vi "BurstVIEW Analysis.vi"() -> ()   [LabVIEW 2017]
uses:
  <vilib>/Utility/config.llb/Config Data RefNum.ctl
  Application/Solution Package/Polarity.ctl
  Application/Solution Package/Minhee Analysis/Minhee analysis parameter_new.ctl
  Application/Solution Package/Data type_new.ctl
  <vilib>/Utility/sysdir.llb/System Directory Type.ctl
  <vilib>/Utility/miscctls.llb/LVRowAndColumnTypeDef.ctl
  <vilib>/Analysis/3filter.llb/Savitzky-Golay Filter (DBL).vi
  <vilib>/Utility/file.llb/Write Delimited Spreadsheet (DBL).vi
  <vilib>/Utility/file.llb/Write Delimited Spreadsheet (string).vi
  <vilib>/Analysis/NI_AALBase.lvlib
  <vilib>/Utility/config.llb/NI_LVConfig.lvlib
panel:
  out "Begin (sec)":string caption="String"
  out "End (sec)":string caption="String"
  out "Frequency":string caption="String"
  out "r^2 =":string caption="String"
  out "Decay t (ms)":string caption="String"
  out "Exponential \ncurve fitting":string
  out "History log":string
  in  "Event Detection Parameter":cluster{"Minimum amplitude":dbl, "Shape":T1}={"Minimum amplitude"=10.0, "Shape"=0} {"Shape" items=["Negative-going", "Positive-going"]}
  in  "Smoothing Parameters":T2={"Polynomial order"=3, "Side points"=35}
  out "Averaged Amplitude":sgl[](graph)
  out "StateFileRefnum":T3
  out "Event":cluster{dbl[], dbl[]}[](graph)
  out "Holding Current":sgl[](graph)
  out "Frequency 2":string caption="String"
  out "Number of event":i32[](graph)
  out "Event # 2":string caption="String"
  out "IEI (sec)  2":string caption="String"
  out "Amplitude 2":string caption="String"
  out "Event #":string caption="String"
  out "IEI (sec)":string caption="String"
  out "Amplitude (pA)":string caption="String"
  in  "Event Num":i16=4 min=0 max=42 step=1
  in  "Sweep Num":u16 max=16 step=1
  out "Event table":string[][](table)
  out "Whole trace":cluster{dbl[], "X":sgl[]}[](graph)
  # "Sweep info."
  # "Event table"
  # "Event detection parameters"
  # "Smoothing parameters"
  # "Result table"
  # "Event #"
  # "Amplitude (pA)"
  # "Total"
  # "IEI (sec)"
  # "Frequency (Hz)"
  # "Event #"
  # "Amplitude (pA)"
  # "IEI (sec)"
  # "Frequency (Hz)"
  # "Selected"
  # "Event search"
  # "Begin (sec)"
  # "End (sec)"
  # "Event"
  # "Sweep"
  # "Sweep"
  # "Log"
  # "(pA)"
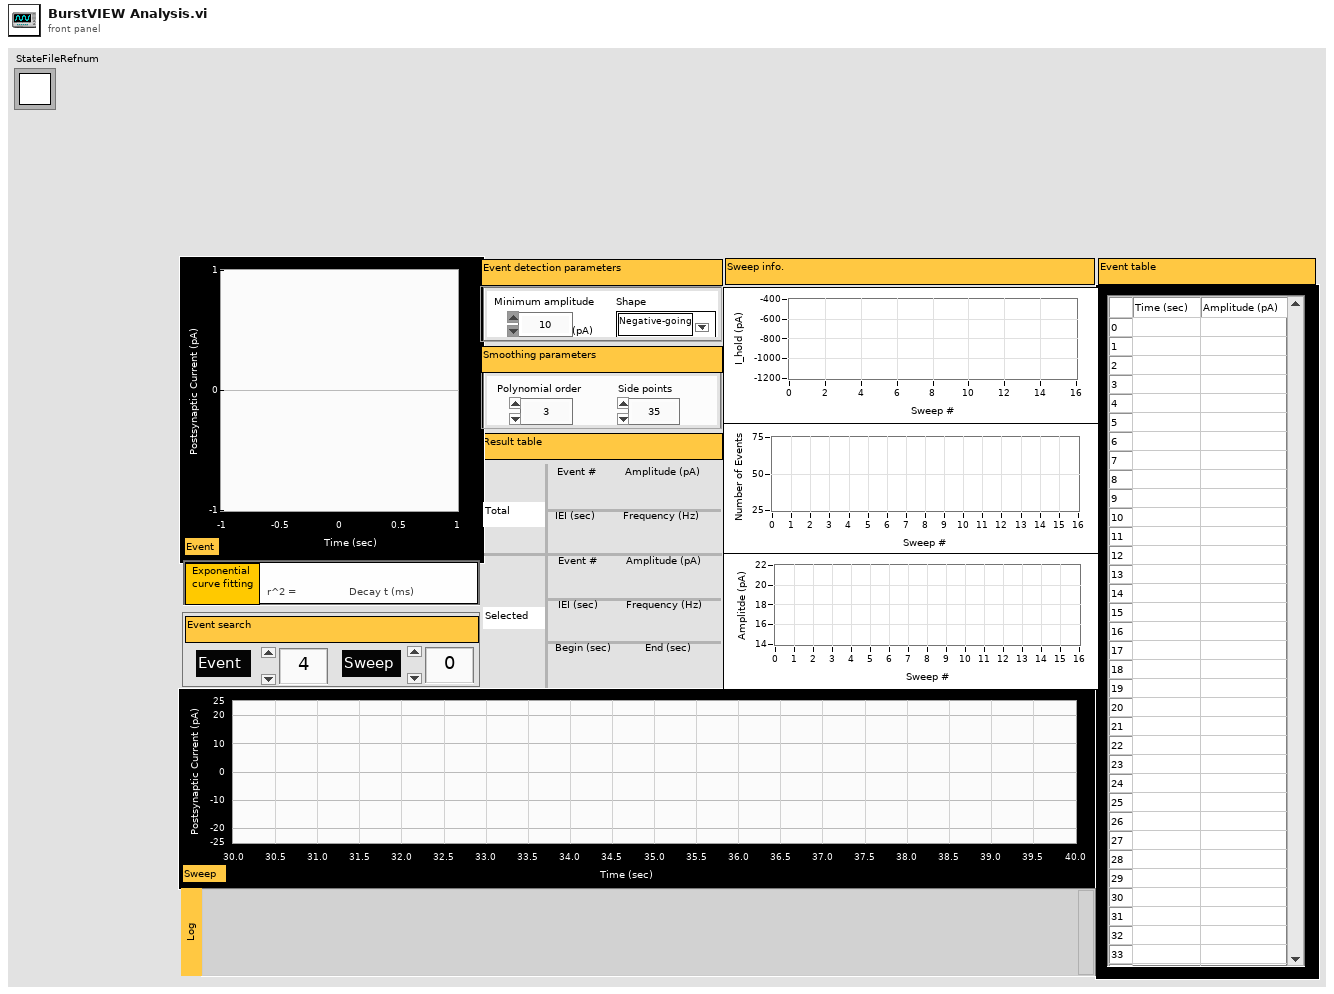
[diagram p1: front panel]
types:
  T1 = typedef "Polarity.ctl" = u16
  T2 = cluster{"Polynomial order":i32, "Side points":i32}
  T3 = typedef "NI_LVConfig.lvlib/Config Data RefNum.ctl" = refnum<k1>
  T4 = enum32{"Invalid", "Standard", "Closed", "Hidden", "Minimized", "Maximized"}
  T5 = enum32{"invalid app kind", "Development System", "Run Time System", "Student Edition", "Embedded LabVIEW", "Evaluation", "Custom"}
  T6 = enum16{"Linear", "Polynomial", "Exponential", "Power"}
  T7 = typedef "Minhee analysis parameter_new.ctl" = cluster{"File":cluster{"File Path":path, "File Name":string, "Total Length":i32, "Trial Length (ms)":dbl, "Sweep Number":dbl, "Sampling rate":dbl, "Data type":T8}, "Smoothing":cluster{"Polynomial order":i32, "Side points":i32}, "Event Detection ":cluster{"Event threshold (amplitude)":dbl, "Polarity":T1}, "Screening":cluster{"Screening threshold (dV/dt)":dbl, " * SD":dbl}}
  T8 = typedef "Data type_new.ctl" = u16
  T9 = cluster{"Core":cluster{"Current VI Reference":refnum<vi>, "Close Panel on Exit?":bool}, "Your Boolean data":bool, "Parameters":T7, "Whole trace (2D)":sgl[][], "Result":cluster{"Sweep Traces (2D)":cluster{sgl[], "X":sgl[]}[][], "Detected Events (1D)":cluster{sgl[][]}[], "Final Baseline":cluster{sgl[][]}[]}, "Running Sweep Num":i32, "Aborted?":bool, "Sweep Info":cluster{"Holding Current":sgl[], "Averaged Amplitude":sgl[], "Number of event":i32[]}, "Number of Event to select":i32, "Sweep Num":u16, "Event Num":i16, "Trace to display":u16, "History log":string, "Summary table":cluster{"Total":cluster{"Event Num":string, "Amplitude":string, "ISI":string, "Frequency":string}, "Selected":cluster{"Event Num":string, "Amplitude":string, "ISI":string, "Frequency":string, "Begin (sec)":string, "End (sec)":string}}, "Smoothing Parameters (1D)":cluster{"Polynomial order":i32, "Side points":i32}[], "Final Data":sgl[][], "Whole Trace selection":u16}
  T10 = cluster{"Polynomial order":i32, "Side points":i32}[]
  T11 = cluster{"Total":cluster{"Event Num":string, "Amplitude":string, "ISI":string, "Frequency":string}, "Selected":cluster{"Event Num":string, "Amplitude":string, "ISI":string, "Frequency":string, "Begin (sec)":string, "End (sec)":string}}
  T12 = cluster{"Sweep Traces (2D)":cluster{sgl[], "X":sgl[]}[][], "Detected Events (1D)":cluster{sgl[][]}[], "Final Baseline":cluster{sgl[][]}[]}
  T13 = cluster{"Holding Current":sgl[], "Averaged Amplitude":sgl[], "Number of event":i32[]}
  T14 = cluster{"Current VI Reference":refnum<vi>, "Close Panel on Exit?":bool}
  T15 = cluster{"Total":cluster{"Event Num":string, "Amplitude":string, "ISI":string, "Frequency":string}, "Selected":cluster{"Event Num":string, "Amplitude":string, "ISI":string, "Frequency":string, "Frequency 2":string, "Frequency 3":string}}
  T16 = typedef "System Directory Type.ctl" = i32
  T17 = typedef "LVRowAndColumnTypeDef.ctl" = cluster{"Row":i32, "Column":i32}
  T18 = cluster{"Event threshold (amplitude)":dbl, "Polarity":T1}
  T19 = cluster{"File Path":path, "Cell ID":string, "File Name":string, "Total Length":i32, "Trial Length (ms)":dbl, "Sweep Number":dbl, "Sampling rate":dbl}
  T20 = typedef "File Parameters.ctl" = cluster{"File path":path, "File name":string, "Total Length":i32, "Trial Length (ms)":i32, "Sweep Number":i32, "Sampling rate":dbl}
  T21 = cluster{"Sampling rate (Hz)":dbl, "Sweep duration (sec)":dbl, "Unit (A or pA)":u16, "Baseline Offset (pA)":dbl}
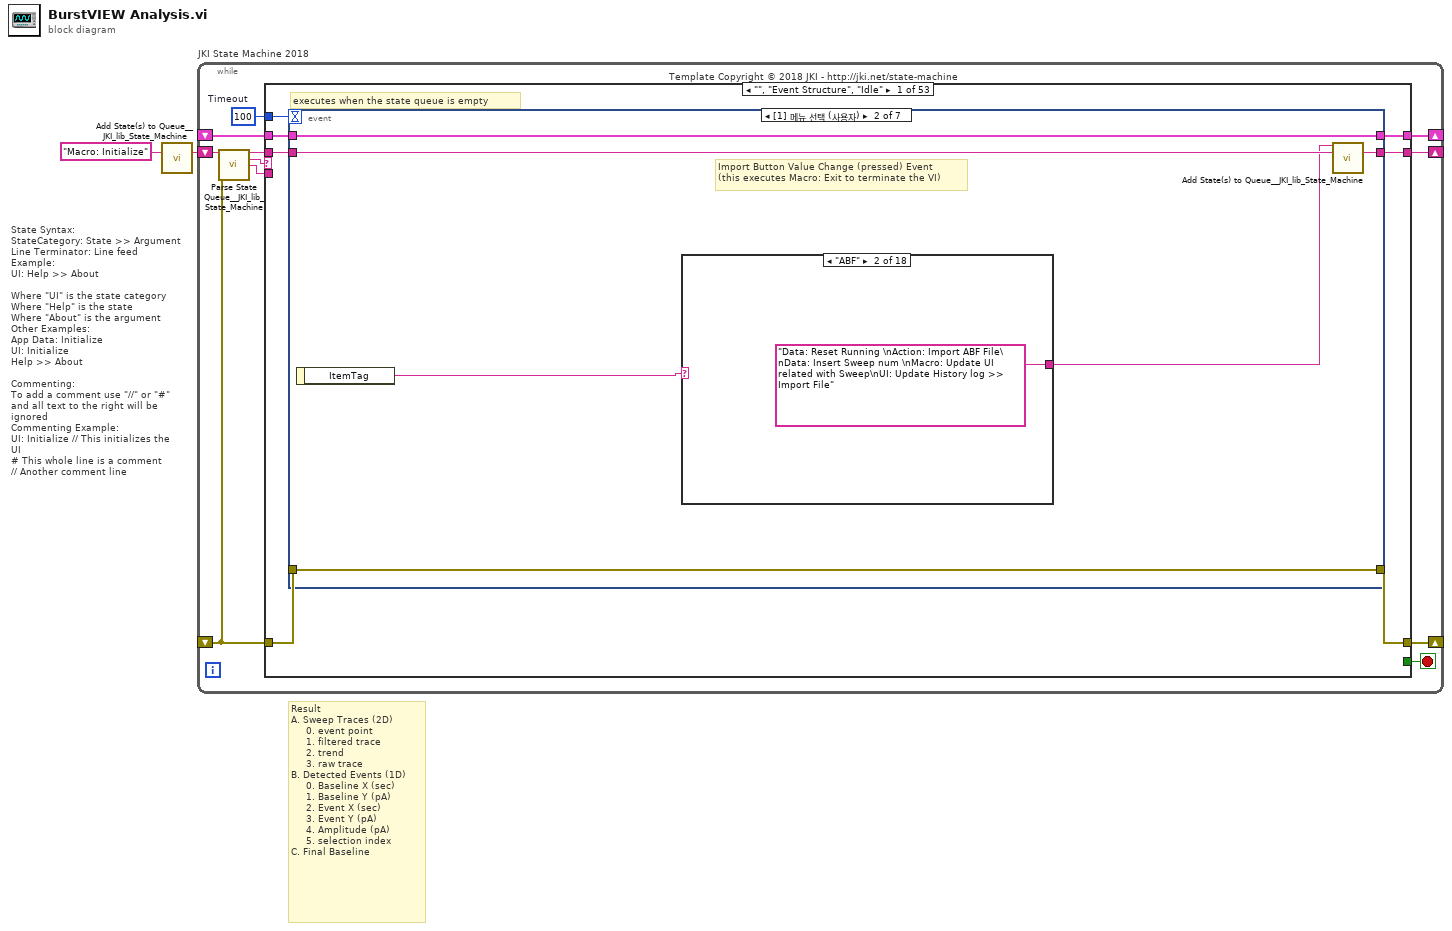
[diagram p0: block diagram]
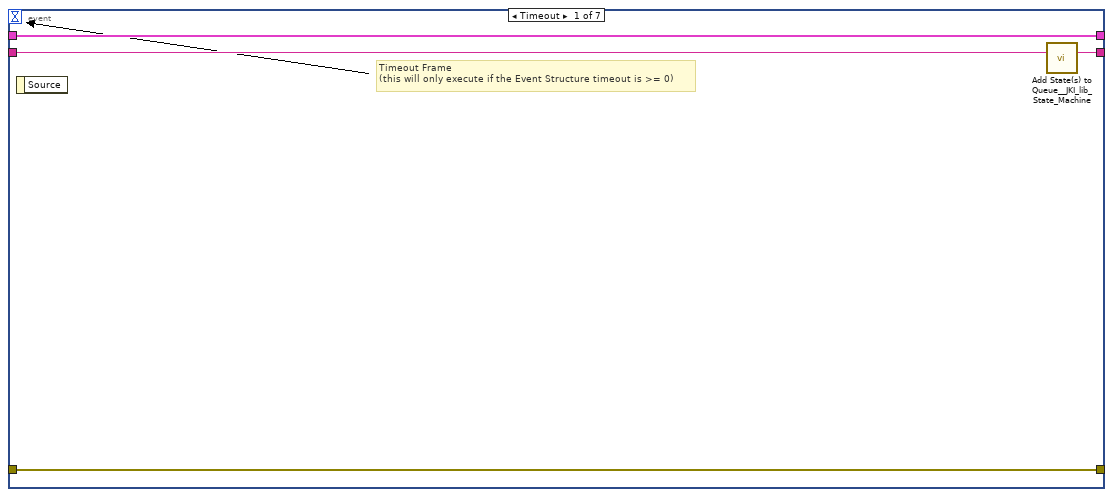
[diagram p2: hidden frame]
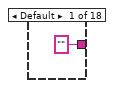
[diagram p3: hidden frame]
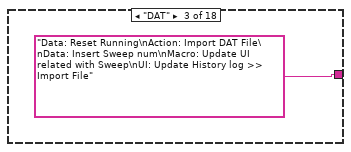
[diagram p4: hidden frame]
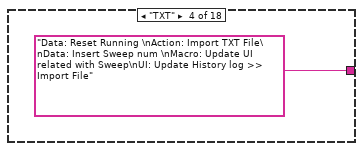
[diagram p5: hidden frame]
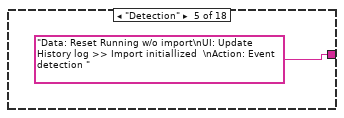
[diagram p6: hidden frame]
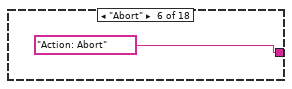
[diagram p7: hidden frame]
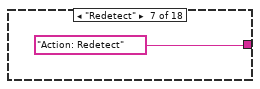
[diagram p8: hidden frame]
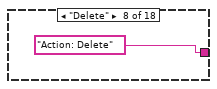
[diagram p9: hidden frame]
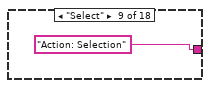
[diagram p10: hidden frame]
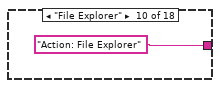
[diagram p11: hidden frame]
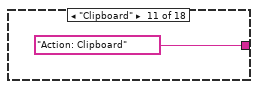
[diagram p12: hidden frame]
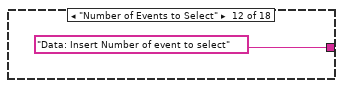
[diagram p13: hidden frame]
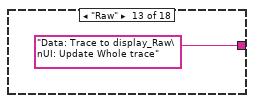
[diagram p14: hidden frame]
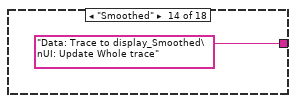
[diagram p15: hidden frame]
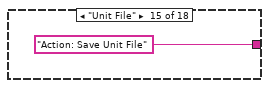
[diagram p16: hidden frame]
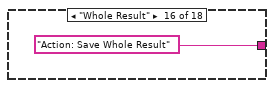
[diagram p17: hidden frame]
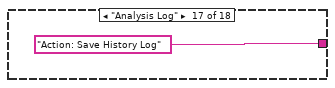
[diagram p18: hidden frame]
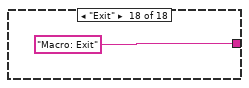
[diagram p19: hidden frame]
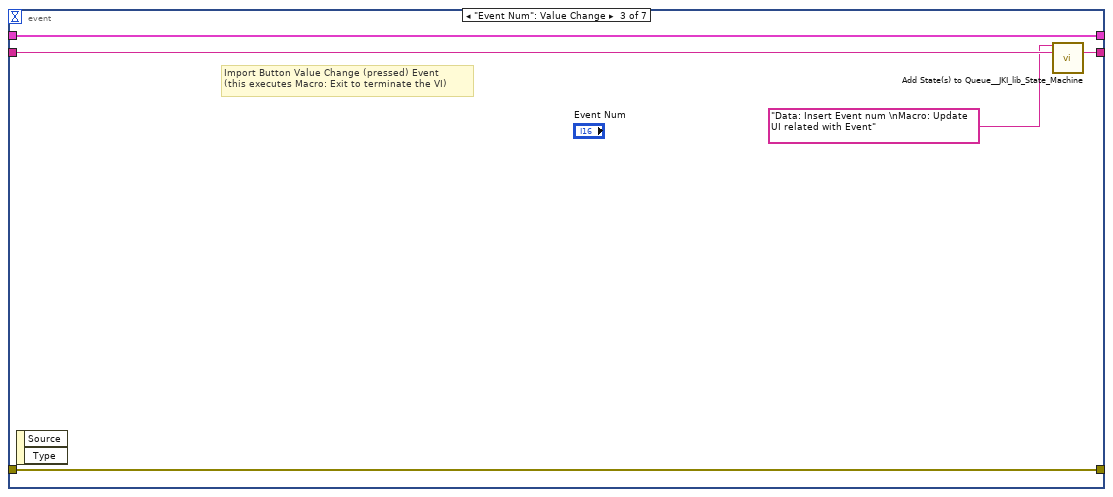
[diagram p20: hidden frame]
diagram:
  # "Result\nA. Sweep Traces (2D)\n     0. event point\n     1. filtered trace\n     2. trend\n     3. raw trace\nB. Detected Events (1D)\n     0. Baseline X (sec)\n     1. Baseline Y (pA)\n     2. Event X (sec)\n     3. Event Y (pA)\n     4. Amplitude (pA)\n     5. selection index\nC. Final Baseline"
  # "State Syntax:\nStateCategory: State >> Argument\nLine Terminator: Line feed\nExample:\nUI: Help >> About\n\nWhere \"UI\" is the state category\nWhere \"Help\" is the state\nWhere \"About\" is the argument\nOther Examples:\nApp Data: Initialize\nUI: Initialize\nHelp >> About\n\nCommenting:\nTo add a comment use \"//\" or \"#\" and all text to the right will be ignored\nCommenting Example:\nUI: Initialize // This initializes the UI\n# This whole line is a comment\n// Another comment line"
  n1 = call <vilib>:"Add State(s) to Queue__JKI_lib_State_Machine.vi"("State(s) in (\"\")"="Macro: Initialize") -> ("States Out"=w2:string)  [unwired: 14 in]
  n2 = while "JKI State Machine 2018" {
    shift-right: [w6] -> _
    shift-left: _ -> [w3]
    shift-right: [w9] -> _
    shift-left: _ -> [w4]
    shift-right: [w8] -> _
    shift-left: w2 -> [w10]
    stop <- w7 stop-if-true
    w5 = 100  # Timeout
    # "Template Copyright © 2018 JKI - http://jki.net/state-machine"
    n3 = call <vilib>:"Parse State Queue__JKI_lib_State_Machine.vi"("State Queue"=w10, "Error In (no error)"=w4) -> ("Remaining States"=w12:string, "Current State"=w13:string, "Arguments"=w11:string)  [unwired: 11 in]
    n4 = case shown="\"\", \"Event Structure\", \"Idle\"" w13 {
      selector: w13 -> [_ _ w79 _ _ _ _ _ _ _ _ _ _ _ _ _ _ _ _ _ _ _ _ _ _ _ _ _ _ _ _ _ _ _ _ _ _ _ _ _ _ _ _ _ _ _ _ _ _ _ _ _ _]
      tunnel: w12 -> [w20 w78 w83 w102 w108 w114 w124 w147 w161 w173 w182 w188 w194 w200 w206 w212 w218 w224 w232 w238 w242 w260 w284 w336 w375 w384 w400 w427 w453 w463 w478 w576 w587 w656 w661 w666 w671 w676 w686 w697 w717 w737 w758 w819 w829 w860 w882 w938 w958 w968 w985 w996 w1005]
      tunnel: w11 -> [_ _ _ _ _ _ _ _ _ _ _ _ _ _ _ _ _ _ _ _ _ _ _ _ _ _ _ _ _ _ w472 w571 w581 _ _ _ _ _ _ _ _ _ _ _ _ _ _ _ _ _ _ _ _]
      tunnel: w3 -> [w18 w75 w81 w95 w105 w112 w121 _ w158 w170 w179 w185 w191 w197 w203 w209 w215 w221 w230 w233 w239 w248 w273 w334 w373 w381 w397 w417 w450 w461 w475 w574 w583 w653 w658 w663 w668 w673 w683 w694 w714 w735 w754 w804 w826 w847 w880 w904 w954 w965 w982 w993 w1002]
      tunnel: [w17 w76 w85 w99 errorcluster {"status"=FALSE, "code"=0, "source"=""} ("error out") w111 w122 w126 w159 w171 w180 w186 w192 w198 w204 w210 w216 w222 w225 w234 w240 w249 w282 w324 w339 w382 w398 w425 w451 w454 w476 w572 w584 w654 w659 w664 w669 w674 w684 w695 w706 w733 w746 w812 w827 w830 w871 w935 w955 w966 w969 w990 w999] -> w9
      tunnel: w4 -> [w16 w76 w84 w99 w104 w111 w122 w127 w159 w171 w180 w186 w192 w198 w204 w210 w216 w222 w226 w235 w240 w246 w267 w325 w340 w382 w398 w425 w451 w455 w476 w573 w585 w654 w659 w664 w669 w674 w684 w695 w699 w728 w756 w813 w827 w831 w872 w935 w956 w966 w970 w991 w1000]
      tunnel: [w19 w77 w82 w101 w107 w113 w123 w146 w160 w172 w181 w187 w193 w199 w205 w211 w217 w223 w231 w237 w241 w259 w283 w335 w374 w383 w399 w426 w452 w462 w477 w575 w586 w655 w660 w665 w670 w675 w685 w696 w716 w736 w757 w818 w828 w859 w881 w937 w957 w967 w984 w995 w1004] -> w8
      tunnel: [_ _ _ _ _ w109 _ _ _ _ _ _ _ _ _ _ _ _ _ _ _ _ _ _ _ _ _ _ _ _ _ _ _ _ _ _ _ _ _ _ _ _ _ _ _ _ _ _ _ _ _ _ _] -> w7
      tunnel: [w15 w75 w81 w100 w105 w112 w121 w145 w157 w169 w178 w184 w190 w196 w202 w208 w214 w220 w229 w233 w239 w248 w273 w334 w373 w381 w397 w416 w450 w461 w474 w574 w583 w653 w658 w663 w668 w673 w683 w694 w713 w734 w753 w803 w825 w846 w879 w903 w954 w965 w982 w993 w1002] -> w6
      tunnel: w5 -> [w14 _ _ _ _ _ _ _ _ _ _ _ _ _ _ _ _ _ _ _ _ _ _ _ _ _ _ _ _ _ _ _ _ _ _ _ _ _ _ _ _ _ _ _ _ _ _ _ _ _ _ _ _]
      frame "", "Event Structure", "Idle" {
        # "executes when the state queue is empty"
        n5 = event shown="[1] 메뉴 선택 (사용자)" {
          selector: _ -> [_ _ _ _ _ _ _]
          dyn-events: _ -> [_ _ _ _ _ _ _]
          timeout: w14 -> [_ _ _ _ _ _ _]
          tunnel: w20 -> [w24 w30 w53 w58 w63 w68 w74]
          tunnel: [w23 w29 w52 w57 w62 w67 w73] -> w19
          tunnel: w18 -> [w21 w27 w49 w54 w59 w64 w71]
          tunnel: [w22 w28 w51 w56 w61 w66 w72] -> w17
          tunnel: w16 -> [w22 w28 w51 w56 w61 w66 w72]
          tunnel: [w21 w27 w49 w54 w59 w64 w71] -> w15
          event Timeout {
            # "Timeout Frame\n(this will only execute if the Event Structure timeout is >= 0)"
            n6 = event-data() -> ()  [unwired: 1 in, 1 out]
            n7 = call <vilib>:"Add State(s) to Queue__JKI_lib_State_Machine.vi"("State(s) in (\"\")"=w24) -> ("States Out"=w23:string)  [unwired: 14 in]
          }
          event Menu Selection (User) {
            # "Import Button Value Change (pressed) Event\n(this executes Macro: Exit to terminate the VI)"
            n8 = event-data() -> ("ItemTag"=w25:string)  [unwired: 1 in]
            n9 = case shown="\"ABF\"" w25 {
              tunnel: ["" "Data: Reset Running \nAction: Import ABF File\nData: Insert Sweep num \nMacro: Update UI related with Sweep\nUI: Update History log >> Import File" "Data: Reset Running\nAction: Import DAT File\nData: Insert Sweep num\nMacro: Update UI related with Sweep\nUI: Update History log >> Import File" "Data: Reset Running \nAction: Import TXT File\nData: Insert Sweep num \nMacro: Update UI related with Sweep\nUI: Update History log >> Import File" "Data: Reset Running w/o import\nUI: Update History log >> Import initiallized  \nAction: Event detection " "Action: Abort" "Action: Redetect" "Action: Delete" "Action: Selection" "Action: File Explorer" "Action: Clipboard" "Data: Insert Number of event to select" "Data: Trace to display_Raw\nUI: Update Whole trace" "Data: Trace to display_Smoothed\nUI: Update Whole trace" "Action: Save Unit File" "Action: Save Whole Result" "Action: Save History Log" "Macro: Exit"] -> w26
              frame Default {
              }
              frame "ABF" {
              }
              frame "DAT" {
              }
              frame "TXT" {
              }
              frame "Detection" {
              }
              frame "Abort" {
              }
              frame "Redetect" {
              }
              frame "Delete" {
              }
              frame "Select" {
              }
              frame "File Explorer" {
              }
              frame "Clipboard" {
              }
              frame "Number of Events to Select" {
              }
              frame "Raw" {
              }
              frame "Smoothed" {
              }
              frame "Unit File" {
              }
              frame "Whole Result" {
              }
              frame "Analysis Log" {
              }
              frame "Exit" {
              }
            }
            n10 = call <vilib>:"Add State(s) to Queue__JKI_lib_State_Machine.vi"("State(s) in Front (\"\")"=w26, "State(s) in (\"\")"=w30) -> ("States Out"=w29:string)  [unwired: 13 in]
          }
          event "Event Num": Value Change {
            # "Import Button Value Change (pressed) Event\n(this executes Macro: Exit to terminate the VI)"
            n11 = event-data() -> ()  [unwired: 1 in, 2 out]
            n12 = call <vilib>:"Add State(s) to Queue__JKI_lib_State_Machine.vi"("State(s) in Front (\"\")"="Data: Insert Event num \nMacro: Update UI related with Event", "State(s) in (\"\")"=w53) -> ("States Out"=w52:string)  [unwired: 13 in]
          }
          event "Sweep Num": Value Change {
            # "Import Button Value Change (pressed) Event\n(this executes Macro: Exit to terminate the VI)"
            n13 = event-data() -> ()  [unwired: 1 in, 2 out]
            n14 = call <vilib>:"Add State(s) to Queue__JKI_lib_State_Machine.vi"("State(s) in Front (\"\")"="Data: Insert Sweep num \nMacro: Update UI related with Sweep \nMacro: Update UI related with Event", "State(s) in (\"\")"=w58) -> ("States Out"=w57:string)  [unwired: 13 in]
          }
          event "Event Detection Parameter.Minimum amplitude": Value Change {
            # "Import Button Value Change (pressed) Event\n(this executes Macro: Exit to terminate the VI)"
            n15 = event-data() -> ()  [unwired: 1 in, 2 out]
            n16 = call <vilib>:"Add State(s) to Queue__JKI_lib_State_Machine.vi"("State(s) in Front (\"\")"="Data: Insert Event detection parameters", "State(s) in (\"\")"=w63) -> ("States Out"=w62:string)  [unwired: 13 in]
          }
          event "Smoothing Parameters.Polynomial order", "Smoothing Parameters.Side points": Value Change {
            # "Import Button Value Change (pressed) Event\n(this executes Macro: Exit to terminate the VI)"
            n17 = event-data() -> ()  [unwired: 1 in, 2 out]
            n18 = call <vilib>:"Add State(s) to Queue__JKI_lib_State_Machine.vi"("State(s) in Front (\"\")"="Data: Insert Smoothing parameters", "State(s) in (\"\")"=w68) -> ("States Out"=w67:string)  [unwired: 13 in]
          }
          event Panel Close? {
            # "Discard the event because we'll close the front panel ourselves in Macro: Exit"
            # "Close Panel button (pressed) Event\n(this executes Macro: Exit to terminate the VI)"
            n19 = event-data() -> ()  [unwired: 1 in, 1 out]
            n20 = call <vilib>:"Add State(s) to Queue__JKI_lib_State_Machine.vi"("State(s) in Front (\"\")"="Macro: Exit", "State(s) in (\"\")"=w74) -> ("States Out"=w73:string)  [unwired: 13 in]
            n21 = event-data("Discard?"=TRUE) -> ()  [unwired: 1 in, 1 out]
          }
        }
      }
      frame "---------- Core ----------" {
        # "Do not put any code in this frame.\n(it is a separator no-op)"
        n22 = call <vilib>:"Add State(s) to Queue__JKI_lib_State_Machine.vi"("State(s) in (\"\")"=w78) -> ("States Out"=w77:string)  [unwired: 14 in]
      }
      frame Default {
        w88 = 42 items=["No error", "Argument error", "Memory is full", "Out of zone", "End of file", "File already open", "Generic file I/O error", "File not found", "File permission error", "Disk is full", "Duplicate path", "Too many files open", "System feature not enabled", "Resource file not found", "Cannot add resource", "Resource not found", "Image not found", "Image memory error", "Pen does not exist", "Config type invalid", "Config token not found", "Config parse error", "Config memory error", "Bad external code format", "Bad external code offset", "External code not present", "Null window", "Destroy window error", "Null menu", "Print aborted", "Bad print record", "Print driver error", "Windows error during printing", "Memory error during printing", "Print dialog error", "Generic print error", "Invalid device refnum", "Device not found", "Device parameter error", "Device unit error", "Cannot open device", "Device call aborted", "Generic error", "Cancelled by user", "Object ID too low", "Object ID too high", "Object not in heap", "Unknown heap", "Unknown object (invalid DefProc)", "Unknown object (DefProc not in table)", "Message out of range", "Invalid (null) method", "Unknown message", "Manager call not supported", "Bad address", "Network operation in progress", "Network operation timed out", "Connection is busy", "Network attribute not supported", "Network error", "Address in use", "System out of memory", "Connection aborted", "Connection refused", "Not connected", "Already connected", "Connection closed", "Initialization error (interapplication manager)", "Bad occurrence", "Wait on unbound occurrence handler", "Occurrence queue overflow", "Datalog type conflict", "Unused", "Unrecognized type (interapplication manager)", "Memory corrupt", "Failed to make temporary DLL", "Old CIN version", "Drag socket not found", "Failed to load drop-object", "Failed to register OLE object", "Failed to release OLE object", "Format specifier type mismatch", "Unknown format specifier", "Too few format specifiers", "Too many format specifiers", "Scan failed", "Newer CIN version", "Error converting to variant", "Runtime menu error", "Password tampered", "Variant attribute not found", "Incompatible variant data type", "Event data is not available", "Event Store is not present", "Occurrence is not found", "Event Queue is not created", "Event info is not available", "Refnum passed is NULL", "Error retrieving Class GUID", "Error retrieving CoClass GUID", "Error retrieving TypeLib GUID.", "Bad built application magic bytes.", "Specific driver is different from the specific driver associated with the Logical Name.", "There is no session opened to the class driver.", "Max Error", "MAX - Error with config objects", "MAX - Error loading configuration", "MAX - Group not supported"]
        # "Current State"
        # "Do not delete, rename, or modify this frame.\n(this is used to capture unhandled states and typos)"
        # "Handle mistyped state name (developer tool)"
        n23 = Format Into String(format string="Software Exception: Unhandled State \"%s\"." ("message"), error in=w84, w79) -> (resulting string=w87:string, error out=w86:errorcluster)  [unwired: 1 in]
        n24 = call <vilib>:"Error Cluster From Error Code.vi"("show call chain? (False)"=TRUE, "error in (no error)"=w86, "error message (\"\")"=w87, "error code (0)"=w88) -> ("error out"=w85:errorcluster)  [unwired: 5 in]
        n25 = call <vilib>:"Add State(s) to Queue__JKI_lib_State_Machine.vi"("State(s) in (\"\")"=w83) -> ("States Out"=w82:string)  [unwired: 14 in]
      }
      frame "Initialize Core Data" {
        # "Do not delete, rename, or modify this frame.\n(this is used to determine panel behavior on exit)"
        # "originally closed?"
        # "exe?"
        # "If panel starts closed or is an EXE, then close it when we exit"
        n26 = property class="VI"() -> ("FP.State"=w92:T4)  [unwired: 2 in, 2 out]
        n27 = property class="App"() -> ("App.Kind"=w98:T5)  [unwired: 2 in, 2 out]
        n28 = control-ref of="Current VI Reference"() -> (w93:refnum<vi>)
        n29 = Equal?(x=w92, y=T4."Closed" ("Front Panel Window:State")) -> (x = y?=w90:bool)
        n30 = Equal?(x=w98, y=T5."Run Time System" ("Application:Kind")) -> (x = y?=w96:bool)
        n31 = Or(x=w90, y=w96) -> (x .or. y?=w94:bool)
        n32 = Bundle By Name(cluster=w95, "Core.Current VI Reference"=w93, "Core.Close Panel on Exit?"=w94) -> (w100:T9)
        n33 = call <vilib>:"Add State(s) to Queue__JKI_lib_State_Machine.vi"("State(s) in (\"\")"=w102) -> ("States Out"=w101:string)  [unwired: 14 in]
      }
      frame "Error Handler" {
        # "Unhandled Error -- Display it"
        # "Handle any errors here.\nYou can also output any states to clean-up after errors occur"
        # "Clear error"
        n34 = call <vilib>:"General Error Handler.vi"("error in (no error)"=w104) -> ()  [unwired: 10 in, 5 out]
        n35 = call <vilib>:"Add State(s) to Queue__JKI_lib_State_Machine.vi"("State(s) in Front (\"\")"="/* Post Error States", "State(s) in (\"\")"=w108) -> ("States Out"=w107:string)  [unwired: 13 in]
      }
      frame "Exit" {
        # "Do not put any code in this frame.\n(No errors that occur here will be handled.)"
        n36 = flat-sequence {
          tunnel: [w115] -> w110
          tunnel: w110 -> [w120]
          tunnel: [w119] -> w109
          frame #0 {
            n37 = local read "StateFileRefnum"() -> (w115:T3)
            n38 = Current VI's Path ("Current VI's Path...")() -> (path=w116:path)
            n39 = Open VI Reference(vi path=w116) -> (vi reference=w117:refnum<vi>)  [unwired: 5 in, 1 out]
            n40 = call <userlib>:"SaveVIState.vi"("StateFileRefnum"=w115, "key"="StateKey", "VI Refnum"=w117) -> ()
          }
          frame #1 {
            w119 = TRUE ("write configuration file? (F)")
            n41 = call <vilib>:"Close Config Data.vi"("write file if changed (T)"=w119, "refnum"=w120) -> ()  [unwired: 8 in, 2 out]
          }
        }
        n42 = call <vilib>:"Add State(s) to Queue__JKI_lib_State_Machine.vi"("State(s) in (\"\")"=w114) -> ("States Out"=w113:string)  [unwired: 14 in]
      }
      frame "---------- Data ----------" {
        # "Do not put any code in this frame.\n(It is a separator no-op. You can make a copy of this frame to create a new Data frame)"
        n43 = call <vilib>:"Add State(s) to Queue__JKI_lib_State_Machine.vi"("State(s) in (\"\")"=w124) -> ("States Out"=w123:string)  [unwired: 14 in]
      }
      frame "Data: Initialize" {
        w125 = u16 0 items=["Imported", "Analyzed"]  # Whole Trace selection
        w131 = sgl[][] []  # Final Data
        w132 = T10 []  # Smoothing Parameters (1D)
        w133 = T11 {"Total"={"Event Num"="", "Amplitude"="", "ISI"="", "Frequency"=""}, "Selected"={"Event Num"="", "Amplitude"="", "ISI"="", "Frequency"="", "Begin (sec)"="", "End (sec)"=""}}  # Summary table
        w134 = ""  # History log
        w135 = u16 0 items=["Raw", "Smoothed"]  # Trace to display
        w136 = T12 {"Sweep Traces (2D)"=[], "Detected Events (1D)"=[], "Final Baseline"=[]}  # Result
        w129 = i16 0  # Event Num
        w130 = u16 0  # Sweep Num
        w137 = 200  # Number of Event to select
        w138 = T13 {"Holding Current"=[], "Averaged Amplitude"=[], "Number of event"=[]}  # Sweep Info
        w139 = FALSE  # Aborted?
        w140 = 0  # Running Sweep Num
        w141 = sgl[][] []  # Whole trace (2D)
        w142 = T7 {"File"={"File Path"=path "", "File Name"="", "Total Length"=0, "Trial Length (ms)"=0.0, "Sweep Number"=0.0, "Sampling rate"=0.0, "Data type"=0}, "Smoothing"={"Polynomial order"=3, "Side points"=20}, "Event Detection "={"Event threshold (amplitude)"=10.0, "Polarity"=0}, "Screening"={"Screening threshold (dV/dt)"=0.0, " * SD"=2.5}}  # Parameters
        w143 = T14 {"Current VI Reference"=refnum, "Close Panel on Exit?"=FALSE}  # Core
        w144 = TRUE  # Your Boolean data
        # "Result\nA. Sweep Traces (2D)\n     0. event point\n     1. filtered trace\n     2. trend\n     3. raw trace\nB. Detected Events (1D)\n     0. Baseline X (sec)\n     1. Baseline Y (pA)\n     2. Event X (sec)\n     3. Event Y (pA)\n     4. Amplitude (pA)\n     5. selection index\nC. Final Baseline"
        # "do not delete - used by framework"
        # "Data names and types of shift register data are defined by this bundle."
        # "Initialize the shift-register data, here.\n(data names are defined by what you wire into the bundle function)"
        n44 = property on="Sweep Num" class="DigNum (엄격한)"(error in=w127, "Value"=w130) -> (error out=w128:errorcluster)  [unwired: 1 in, 1 out]
        n45 = property on="Event Num" class="DigNum (엄격한)"(error in=w128, "Value"=w129) -> (error out=w126:errorcluster)  [unwired: 1 in, 1 out]
        n46 = Bundle("Core"=w143, "Your Boolean data"=w144, "Parameters"=w142, "Whole trace (2D)"=w141, "Result"=w136, "Running Sweep Num"=w140, "Aborted?"=w139, "Sweep Info"=w138, "Number of Event to select"=w137, "Sweep Num"=w130, "Event Num"=w129, "Trace to display"=w135, "History log"=w134, "Summary table"=w133, "Smoothing Parameters (1D)"=w132, "Final Data"=w131, "Whole Trace selection"=w125) -> (w145:T9)  [unwired: 1 in]
        n47 = call <vilib>:"Add State(s) to Queue__JKI_lib_State_Machine.vi"("State(s) in (\"\")"=w147) -> ("States Out"=w146:string)  [unwired: 14 in]
      }
      frame "Data: Reset Running" {
        w148 = u16 0 items=["Imported", "Analyzed"]  # Whole Trace selection
        w151 = T15 {"Total"={"Event Num"="", "Amplitude"="", "ISI"="", "Frequency"=""}, "Selected"={"Event Num"="", "Amplitude"="", "ISI"="", "Frequency"="", "Frequency 2"="", "Frequency 3"=""}}  # Summary table
        w152 = T12 {"Sweep Traces (2D)"=[], "Detected Events (1D)"=[], "Final Baseline"=[]}  # Result
        w154 = T13 {"Holding Current"=[], "Averaged Amplitude"=[], "Number of event"=[]}  # Sweep Info
        # "Do not put any code in this frame.\n(It is a separator no-op. You can make a copy of this frame to create a new Data frame)"
        n48 = Bundle By Name(cluster=w158, "Running Sweep Num"=0 ("Running Sweep #"), "Aborted?"=FALSE ("Aborted"), "Sweep Info"=w154, "Whole trace (2D)"=sgl[][] [], "Result"=w152, "Summary table"=w151, "Whole Trace selection"=w148) -> (w157:T9)
        n49 = local write "Whole trace"(cluster{sgl[], "X":sgl[]}[] [{[], "X"=[]}, {[], "X"=[]}, {[], "X"=[]}] ("Whole trace")) -> ()
        n50 = local write "Event"(cluster{sgl[], sgl[]}[] [{[], []}, {[], []}, {[], []}, {[], []}] ("Event trace")) -> ()
        n51 = call <vilib>:"Add State(s) to Queue__JKI_lib_State_Machine.vi"("State(s) in (\"\")"=w161) -> ("States Out"=w160:string)  [unwired: 14 in]
      }
      frame "Data: Reset Running w/o import" {
        w164 = T15 {"Total"={"Event Num"="", "Amplitude"="", "ISI"="", "Frequency"=""}, "Selected"={"Event Num"="", "Amplitude"="", "ISI"="", "Frequency"="", "Frequency 2"="", "Frequency 3"=""}}  # Summary table
        w165 = T12 {"Sweep Traces (2D)"=[], "Detected Events (1D)"=[], "Final Baseline"=[]}  # Result
        w166 = T13 {"Holding Current"=[], "Averaged Amplitude"=[], "Number of event"=[]}  # Sweep Info
        # "Do not put any code in this frame.\n(It is a separator no-op. You can make a copy of this frame to create a new Data frame)"
        n52 = Bundle By Name(cluster=w170, "Running Sweep Num"=0 ("Running Sweep #"), "Aborted?"=FALSE ("Aborted"), "Sweep Info"=w166, "Result"=w165, "Summary table"=w164) -> (w169:T9)
        n53 = local write "Whole trace"(cluster{sgl[], "X":sgl[]}[] [{[], "X"=[]}, {[], "X"=[]}, {[], "X"=[]}] ("Whole trace")) -> ()
        n54 = local write "Event"(cluster{sgl[], sgl[]}[] [{[], []}, {[], []}, {[], []}, {[], []}] ("Event trace")) -> ()
        n55 = call <vilib>:"Add State(s) to Queue__JKI_lib_State_Machine.vi"("State(s) in (\"\")"=w173) -> ("States Out"=w172:string)  [unwired: 14 in]
      }
      frame "Data: Insert inital parameters" {
        # "Do not put any code in this frame.\n(It is a separator no-op. You can make a copy of this frame to create a new Data frame)"
        n56 = local read "Event Detection Parameter"() -> (w175:cluster{"Minimum amplitude":dbl, "Shape":T1})
        n57 = local read "Smoothing Parameters"() -> (w174:T2)
        n58 = local read "Sweep Num"() -> (w177:u16)
        n59 = local read "Event Num"() -> (w176:i16)
        n60 = Bundle By Name(cluster=w179, "Sweep Num"=w177, "Event Num"=w176, "Parameters.Smoothing"=w174, "Parameters.Event Detection"=w175) -> (w178:T9)
        n61 = call <vilib>:"Add State(s) to Queue__JKI_lib_State_Machine.vi"("State(s) in (\"\")"=w182) -> ("States Out"=w181:string)  [unwired: 14 in]
      }
      frame "Data: Insert Sweep num" {
        # "Do not put any code in this frame.\n(It is a separator no-op. You can make a copy of this frame to create a new Data frame)"
        n62 = local read "Sweep Num"() -> (w183:u16)
        n63 = Bundle By Name(cluster=w185, "Sweep Num"=w183) -> (w184:T9)
        n64 = call <vilib>:"Add State(s) to Queue__JKI_lib_State_Machine.vi"("State(s) in (\"\")"=w188) -> ("States Out"=w187:string)  [unwired: 14 in]
      }
      frame "Data: Insert Event num" {
        # "Do not put any code in this frame.\n(It is a separator no-op. You can make a copy of this frame to create a new Data frame)"
        n65 = local read "Event Num"() -> (w189:i16)
        n66 = Bundle By Name(cluster=w191, "Event Num"=w189) -> (w190:T9)
        n67 = call <vilib>:"Add State(s) to Queue__JKI_lib_State_Machine.vi"("State(s) in (\"\")"=w194) -> ("States Out"=w193:string)  [unwired: 14 in]
      }
      frame "Data: Insert Event detection parameters" {
        # "Do not put any code in this frame.\n(It is a separator no-op. You can make a copy of this frame to create a new Data frame)"
        n68 = local read "Event Detection Parameter"() -> (w195:cluster{"Minimum amplitude":dbl, "Shape":T1})
        n69 = Bundle By Name(cluster=w197, "Parameters.Event Detection"=w195) -> (w196:T9)
        n70 = call <vilib>:"Add State(s) to Queue__JKI_lib_State_Machine.vi"("State(s) in (\"\")"=w200) -> ("States Out"=w199:string)  [unwired: 14 in]
      }
      frame "Data: Insert Smoothing parameters" {
        n71 = local read "Smoothing Parameters"() -> (w201:T2)
        n72 = Bundle By Name(cluster=w203, "Parameters.Smoothing"=w201) -> (w202:T9)
        n73 = call <vilib>:"Add State(s) to Queue__JKI_lib_State_Machine.vi"("State(s) in (\"\")"=w206) -> ("States Out"=w205:string)  [unwired: 14 in]
      }
      frame "Data: Trace to display_Raw" {
        # "Do not put any code in this frame.\n(It is a separator no-op. You can make a copy of this frame to create a new Data frame)"
        n74 = Bundle By Name(cluster=w209, "Trace to display"=u16 0) -> (w208:T9)
        n75 = call <vilib>:"Add State(s) to Queue__JKI_lib_State_Machine.vi"("State(s) in (\"\")"=w212) -> ("States Out"=w211:string)  [unwired: 14 in]
      }
      frame "Data: Trace to display_Smoothed" {
        # "Do not put any code in this frame.\n(It is a separator no-op. You can make a copy of this frame to create a new Data frame)"
        n76 = Bundle By Name(cluster=w215, "Trace to display"=u16 1) -> (w214:T9)
        n77 = call <vilib>:"Add State(s) to Queue__JKI_lib_State_Machine.vi"("State(s) in (\"\")"=w218) -> ("States Out"=w217:string)  [unwired: 14 in]
      }
      frame "Data: Whole trace selection" {
        # "Do not put any code in this frame.\n(It is a separator no-op. You can make a copy of this frame to create a new Data frame)"
        n78 = Bundle By Name(cluster=w221, "Whole Trace selection"=u16 1) -> (w220:T9)
        n79 = call <vilib>:"Add State(s) to Queue__JKI_lib_State_Machine.vi"("State(s) in (\"\")"=w224) -> ("States Out"=w223:string)  [unwired: 14 in]
      }
      frame "Data: Insert Number of event to select" {
        # "Do not put any code in this frame.\n(It is a separator no-op. You can make a copy of this frame to create a new Data frame)"
        n80 = call "Number of Events to Select"("error in (no error)"=w226) -> ("Number of Events"=w228:dbl, "error out"=w225:errorcluster)  [unwired: 16 in, 1 out]
        n81 = To Long Integer(number=w228) -> (32bit integer=w227:i32)
        n82 = Bundle By Name(cluster=w230, "Number of Event to select"=w227) -> (w229:T9)
        n83 = call <vilib>:"Add State(s) to Queue__JKI_lib_State_Machine.vi"("State(s) in (\"\")"=w232) -> ("States Out"=w231:string)  [unwired: 14 in]
      }
      frame "Data: Cleanup" {
        # "Cleanup any data and references, here.\n(this is called automatically, by the Macro: Exit)"
        n84 = Unbundle By Name(w233) -> ("Core.Current VI Reference"=w236:refnum<vi>)
        n85 = Close Reference(reference=w236, error in (no error)=w235) -> (error out=w234:errorcluster)
        n86 = call <vilib>:"Add State(s) to Queue__JKI_lib_State_Machine.vi"("State(s) in (\"\")"=w238) -> ("States Out"=w237:string)  [unwired: 14 in]
      }
      frame "---------- UI ----------" {
        # "Do not put any code in this frame.\n(It is a separator no-op. You can make a copy of this frame to create a new UI frame)"
        n87 = call <vilib>:"Add State(s) to Queue__JKI_lib_State_Machine.vi"("State(s) in (\"\")"=w242) -> ("States Out"=w241:string)  [unwired: 14 in]
      }
      frame "UI: Initialize" {
        w256 = T16 6 items=["사용자 홈"=0, "사용자 데스크탑"=1, "사용자 문서"=2, "사용자 어플리케이션 데이터"=3, "사용자 환경"=4, "사용자 임시"=5, "퍼블릭 문서"=6, "퍼블릭 어플리케이션 데이터"=7, "퍼블릭 환경"=8, "퍼블릭 캐시"=13, "시스템 코어 라이브러리"=9, "시스템 설치된 라이브러리"=10, "어플리케이션 파일"=11, "부팅 볼륨 루트"=12] ("system directory type")
        # "Initialize the User Interface, here.\n(this is called automatically, by the Macro: Init)"
        n88 = Unbundle By Name(w248) -> ("Core.Current VI Reference"=w247:refnum<vi>)
        n89 = property class="VI"(reference=w247, error in=w246, "Front Panel.Title"="BurstVIEW Analysis (0.1.0)" ("프런트패널 윈도우:제목"), "Front Panel.Resizeable"=FALSE ("프런트패널 윈도우:크기 조정 가능")) -> (error out=w245:errorcluster)  [unwired: 1 out]
        n90 = call <userlib>:"Default folder.vi"("Folder name"="BurstVIEW Analysis Pack", "system directory type"=w256) -> ("Folder path"=w258:path)  [unwired: 5 in]
        n91 = Current VI's Path ("Current VI Path...")() -> (path=w254:path)
        n92 = Build Path(base path=w258, name or relative path="BurstVIEW Analysis.ini") -> (appended path=w251:path)
        n93 = Open VI Reference(vi path=w254, error in (no error)=w245) -> (vi reference=w253:refnum<vi>, error out=w249:errorcluster)  [unwired: 4 in]
        n94 = call <userlib>:"InitializeStateFile.vi"("key"="StateKey", "configuration file path"=w251, "VI Refnum"=w253) -> ("StateFileRefnum"=→"StateFileRefnum":T3)
        n95 = call <vilib>:"Add State(s) to Queue__JKI_lib_State_Machine.vi"("State(s) in (\"\")"=w260) -> ("States Out"=w259:string)  [unwired: 14 in]
      }
      frame "UI: Update Whole trace" {
        n96 = Unbundle By Name(w273) -> ("Whole trace (2D)"=w265:sgl[][], "Result.Sweep Traces (2D)"=w271:cluster{sgl[], "X":sgl[]}[][], "Sweep Num"=w270:u16, "Trace to display"=w269:u16, "Sweep Info.Number of event"=w268:i32[], "Parameters.File.Trial Length (ms)"=w264:dbl, "Parameters.File.Sampling rate"=w263:dbl, "Whole Trace selection"=w261:u16)
        n97 = case shown="1, 기본" w261 {
          tunnel: [w288 w310] -> w272
          tunnel: w271 -> [_ w309]
          tunnel: w270 -> [w294 w308]
          tunnel: w269 -> [_ w307]
          tunnel: w268 -> [_ w306]
          tunnel: w267 -> [w286 w305]
          tunnel: [w286 w303] -> w266
          tunnel: w265 -> [w297 _]
          tunnel: w264 -> [w296 _]
          tunnel: w263 -> [w293 _]
          tunnel: [w287 w302] -> w262
          frame 0 {
            # "Imported trace"
            n98 = Divide(x=w296, y=w293) -> (x/y=w295:dbl)
            n99 = Index Array(array=w297, index (row)=w294) -> (element=w287:sgl[])  [unwired: 1 in]
            n100 = Multiply(x=w294, y=w295) -> (x*y=w291:dbl)
            n101 = for {
              tunnel: w287 -> [_] mode=indexing
              tunnel: w293 -> [w301]
              tunnel: [w298] -> w292 mode=indexing
              i -> [w299]
              n102 = Reciprocal(x=w301) -> (1/x=w300:dbl)
              n103 = Multiply(x=w300, y=w299) -> (x*y=w298:dbl)
            }
            n104 = Add(x=w291, y=w292) -> (x+y=w290:dbl[])
            n105 = Bundle(w290, "Whole trace (2D)"=w287) -> (w289:cluster{dbl[], "Whole trace (2D)":sgl[]})  [unwired: 1 in]
            n106 = Build Array(cluster{dbl[], "Whole trace (2D)":sgl[]} {[], "Whole trace (2D)"=[]} ("원소"), w289) -> (w288:cluster{dbl[], "Whole trace (2D)":sgl[]}[])
          }
          frame 1, Default {
            # "Analyzed trace"
            # "0 raw trace\n1 filtered trace"
            n107 = Index Array(array=w306, index=w308) -> (element=w320:i32)
            n108 = Index Array(array=w309, index (row)=w308) -> (element=w315:cluster{sgl[], "X":sgl[]}[])  [unwired: 1 in]
            n109 = Decrement(x=w320) -> (x-1=w321:i32)
            n110 = Index Array(array=w315, index #1=0 ("인덱스"), index #2=1 ("인덱스"), index #3=2 ("인덱스")) -> (element #1=w316:cluster{sgl[], "X":sgl[]}, element #2=w319:cluster{sgl[], "X":sgl[]}, element #3=w317:cluster{sgl[], "X":sgl[]}, element #4=w304:cluster{sgl[], "X":sgl[]})  [unwired: 1 in]
            n111 = case shown="0, 기본" w307 {
              tunnel: w319 -> [_ w323]
              tunnel: [w322 w323] -> w318
              tunnel: w304 -> [w322 _]
              frame 0, Default {
              }
              frame 1 {
              }
            }
            n112 = property on="Event Num" class="DigNum (엄격한)"(error in=w305, "Maximum"=w321, "Minimum"=0.0 ("데이터 입력 제한:최소")) -> (error out=w303:errorcluster)  [unwired: 1 in, 1 out]
            n113 = Build Array(w316, w318, w317) -> (w310:cluster{sgl[], "X":sgl[]}[])
            n114 = Unbundle By Name(w304) -> ("X"=w302:sgl[])
          }
        }
        "Whole trace" <- w272
        n115 = Array Max & Min(array=w262) -> (max value=w281:sgl, min value=w280:sgl)  [unwired: 2 out]
        n116 = Add(x=w281, y=25.0 ("x")) -> (x+y=w279:dbl)
        n117 = Add(x=w280, y=-25.0 ("x")) -> (x+y=w276:dbl)
        n118 = Round Toward +Infinity(x=w279) -> (ceil(x): smallest int >= x=w278:dbl)
        n119 = Round Toward +Infinity(x=w276) -> (ceil(x): smallest int >= x=w277:dbl)
        n120 = property on="Whole trace" class="XYGraph (엄격한)"(error in=w266, "YScale.Minimum"=w277, "YScale.Maximum"=w278) -> (error out=w282:errorcluster)  [unwired: 1 in, 1 out]
        n121 = call <vilib>:"Add State(s) to Queue__JKI_lib_State_Machine.vi"("State(s) in (\"\")"=w284) -> ("States Out"=w283:string)  [unwired: 14 in]
      }
      frame "UI: Update Whole trace cursor" {
        # "Do not put any code in this frame.\n(It is a separator no-op. You can make a copy of this frame to create a new UI frame)"
        n122 = Unbundle By Name(w334) -> ("Result.Detected Events (1D)"=w333:cluster{sgl[][]}[], "Sweep Num"=w332:u16, "Event Num"=w329:i16)
        n123 = Index Array(array=w333, index=w332) -> (element=w331:cluster{sgl[][]})
        n124 = Unbundle(w331) -> (w330:sgl[][])
        n125 = Index Array(array=w330, index (row)=w329) -> (element=w328:sgl[])  [unwired: 1 in]
        n126 = Index Array(array=w328) -> (element=w327:sgl)  [unwired: 1 in]
        n127 = property on="Whole trace" class="XYGraph (엄격한)"(error in=w325, "Active Cursor"=u32 0 ("활성 커서"), "Cursor.Cursor X"=w327) -> (error out=w324:errorcluster)  [unwired: 1 in, 1 out]
        n128 = call <vilib>:"Add State(s) to Queue__JKI_lib_State_Machine.vi"("State(s) in (\"\")"=w336) -> ("States Out"=w335:string)  [unwired: 14 in]
      }
      frame "UI: Update Event trace" {
        w358 = T17 {"Row"=0, "Column"=0} ("선택 시작")
        # "Do not put any code in this frame.\n(It is a separator no-op. You can make a copy of this frame to create a new UI frame)"
        n129 = Unbundle By Name(w373) -> ("Parameters.File.Sampling rate"=w369:dbl, "Result.Detected Events (1D)"=w371:cluster{sgl[][]}[], "Result.Sweep Traces (2D)"=w372:cluster{sgl[], "X":sgl[]}[][], "Sweep Num"=w370:u16, "Event Num"=w355:i16, "Parameters.File.Data type"=w366:T8, "Parameters.Event Detection.Polarity"=w367:T1)  [unwired: 1 out]
        n130 = Reciprocal(x=w369) -> (1/x=w368:dbl)
        n131 = call "Update Event trace.vi"("Event Detection Parameter.Polarity"=w367, "dt"=w368, "Data type"=w366, "Event #"=w355, "Sweep #"=w370, "Sweep trace (2D) In"=w372, "Detected Event (1D) In"=w371) -> ("SSE, R^2, RMSE"=w347:dbl[], "best fit parameters"=w344:dbl[], "event"=→"Event":cluster{dbl[], dbl[]}[])  [unwired: 2 in]
        n132 = Number To Fractional String(number=w347, precision (6)=i16 2 ("정밀도(6)")) -> (F-format string=w349:string[])  [unwired: 2 in]
        n133 = Subtract(x=w355, y=35) -> (x-y=w353:i32)
        n134 = Index Array(array=w349, index #1=1 ("인덱스"), index #2=3 ("인덱스")) -> (element #1=→"r^2 =":string, element #2=→"Decay t (ms)":string)  [unwired: 1 in, 1 out]
        n135 = Greater Or Equal To 0?(x=w353) -> (x >= 0?=w354:bool)
        n136 = case shown="거짓" w354 {
          tunnel: w353 -> [_ w377]
          tunnel: [0 w377] -> w352
          frame False {
          }
          frame True {
          }
        }
        n137 = call "Regression Equation String.vi"("coefficients"=w344, "precision"=2, "fit type"=T6."Exponential") -> ("Formula"=w342:string)  [unwired: 8 in]
        n138 = Bundle(cluster=w358, "Row"=w355, "Column"=u32 0 ("활성 커서")) -> (w359:T17)
        n139 = Bundle(cluster=w358, "Row"=u32 1 ("활성 커서"), "Column"=u32 2 ("활성 커서")) -> (w363:T17)
        n140 = Bundle By Name(cluster=w358, "Row"=w352) -> (w357:T17)
        n141 = Concatenate Strings("y = " ("string"), w342) -> (→"Exponential \ncurve fitting":string)
        n142 = property on="Event table" class="Tbl (엄격한)"(error in=w340, "Selection Start"=w359, "Selection Size"=w363, "Selection Color"=u32 15704576, "Index Values"=w357) -> (error out=w339:errorcluster)  [unwired: 1 in, 1 out]
        n143 = call <vilib>:"Add State(s) to Queue__JKI_lib_State_Machine.vi"("State(s) in (\"\")"=w375) -> ("States Out"=w374:string)  [unwired: 14 in]
      }
      frame "UI: Update Sweep Info" {
        # "Do not put any code in this frame.\n(It is a separator no-op. You can make a copy of this frame to create a new UI frame)"
        n144 = Unbundle By Name(w381) -> ("Sweep Info.Holding Current"=→"Holding Current":sgl[], "Sweep Info.Averaged Amplitude"=→"Averaged Amplitude":sgl[], "Sweep Info.Number of event"=→"Number of event":i32[])
        n145 = call <vilib>:"Add State(s) to Queue__JKI_lib_State_Machine.vi"("State(s) in (\"\")"=w384) -> ("States Out"=w383:string)  [unwired: 14 in]
      }
      frame "UI: Update Event Table" {
        # "0. Baseline X (sec)\n1. Baseline Y (pA)\n2. Event X (sec)\n3. Event Y (pA)\n4. Amplitude (pA)\n5. selection index"
        # "Do not put any code in this frame.\n(It is a separator no-op. You can make a copy of this frame to create a new UI frame)"
        n146 = Unbundle By Name(w397) -> ("Result.Detected Events (1D)"=w390:cluster{sgl[][]}[], "Sweep Num"=w389:u16)
        n147 = Index Array(array=w390, index=w389) -> (element=w388:cluster{sgl[][]})
        n148 = Unbundle(w388) -> (w391:sgl[][])
        n149 = Index Array(array=w391, index (col) #1=0 ("비활성화된 인덱스 (열)"), index (col) #2=4 ("인덱스 (열)")) -> (element #1=w395:sgl[], element #2=w396:sgl[])  [unwired: 2 in]
        n150 = Build Array(w395, w396) -> (w387:sgl[][])
        n151 = Transpose 2D Array(2D array=w387) -> (transposed array=w386:sgl[][])
        n152 = Number To Fractional String(number=w386, precision (6)=i16 3 ("폭(-)")) -> (F-format string=→"Event table":string[][])  [unwired: 2 in]
        n153 = call <vilib>:"Add State(s) to Queue__JKI_lib_State_Machine.vi"("State(s) in (\"\")"=w400) -> ("States Out"=w399:string)  [unwired: 14 in]
      }
      frame "UI: Update Total table" {
        w406 = sgl[] []
        # "Do not put any code in this frame.\n(It is a separator no-op. You can make a copy of this frame to create a new UI frame)"
        n154 = Unbundle By Name(w417) -> ("Result.Detected Events (1D)"=w413:cluster{sgl[][]}[], "Sweep Info.Number of event"=w424:i32[], "Parameters.File.Total Length"=w423:i32, "Parameters.File.Sampling rate"=w422:dbl)
        n155 = for {
          tunnel: w413 -> [w441] mode=indexing
          shift-right: [w438] -> w408
          shift-left: w406 -> [w437]
          shift-right: [w435] -> w403
          shift-left: w406 -> [w434]
          n156 = Unbundle(w441) -> (w440:sgl[][])
          n157 = Index Array(array=w440, index (col) #1=4 ("비활성화된 인덱스 (열)"), index (col) #2=2 ("인덱스 (열)")) -> (element #1=w439:sgl[], element #2=w436:sgl[])  [unwired: 2 in]
          n158 = Insert Into Array(array=w437, new element=w439) -> (w438:sgl[])  [unwired: 1 in]
          n159 = Insert Into Array(array=w434, new element=w436) -> (w435:sgl[])  [unwired: 1 in]
        }
        n160 = Divide(x=w423, y=w422) -> (x/y=w420:dbl)
        n161 = Add Array Elements(numeric array=w424) -> (sum=w421:i32)
        n162 = Divide(x=w421, y=w420) -> (x/y=w419:dbl)
        n163 = Number To Decimal String(number=w421) -> (decimal integer string=w414:string)  [unwired: 1 in]
        "Event #" <- w414
        n164 = Number To Fractional String(number=w419, precision (6)=i16 3 ("정밀도(6)")) -> (F-format string=w415:string)  [unwired: 2 in]
        "Frequency" <- w415
        n165 = call <vilib>:"Std Deviation and Variance.vi"("X"=w408) -> ("mean"=w407:dbl)  [unwired: 1 in, 2 out]
        n166 = Array Size(array=w403) -> (size(s)=w405:i32)
        n167 = Decrement(x=w405) -> (x-1=w404:i32)
        n168 = Number To Fractional String(number=w407, precision (6)=i16 2 ("폭(-)")) -> (F-format string=w402:string)  [unwired: 2 in]
        "Amplitude (pA)" <- w402
        n169 = for {
          N: w404 -> [_]
          tunnel: [w431] -> w410 mode=indexing
          tunnel: w403 -> [w430]
          i -> [w432]
          n170 = Increment(x=w432) -> (x+1=w433:i32)
          n171 = Index Array(array=w430, index #1=w433, index #2=w432) -> (element #1=w429:sgl, element #2=w428:sgl)
          n172 = Subtract(x=w429, y=w428) -> (x-y=w431:sgl)
        }
        n173 = call <vilib>:"Std Deviation and Variance.vi"("X"=w410) -> ("mean"=w412:dbl)  [unwired: 1 in, 2 out]
        n174 = Number To Fractional String(number=w412, precision (6)=i16 2 ("폭(-)")) -> (F-format string=w401:string)  [unwired: 2 in]
        "IEI (sec)" <- w401
        n175 = Bundle By Name(cluster=w417, "Summary table.Total.Event Num"=w414, "Summary table.Total.Frequency"=w415, "Summary table.Total.Amplitude"=w402, "Summary table.Total.ISI"=w401) -> (w416:T9)
        n176 = call <vilib>:"Add State(s) to Queue__JKI_lib_State_Machine.vi"("State(s) in (\"\")"=w427) -> ("States Out"=w426:string)  [unwired: 14 in]
      }
      frame "UI: Update Selected table" {
        # "Do not put any code in this frame.\n(It is a separator no-op. You can make a copy of this frame to create a new UI frame)"
        n177 = Unbundle By Name(w450) -> ("Summary table.Selected.Event Num"=→"Event # 2":string, "Summary table.Selected.Amplitude"=→"Amplitude 2":string, "Summary table.Selected.ISI"=→"IEI (sec)  2":string, "Summary table.Selected.Frequency"=→"Frequency 2":string, "Summary table.Selected.Begin (sec)"=→"Begin (sec)":string, "Summary table.Selected.End (sec)"=→"End (sec)":string)
        n178 = call <vilib>:"Add State(s) to Queue__JKI_lib_State_Machine.vi"("State(s) in (\"\")"=w453) -> ("States Out"=w452:string)  [unwired: 14 in]
      }
      frame "UI: Update Sweep infor cursor" {
        w459 = u32 0 ("활성 커서")
        # "Do not put any code in this frame.\n(It is a separator no-op. You can make a copy of this frame to create a new UI frame)"
        n179 = Unbundle By Name(w461) -> ("Sweep Num"=w460:u16)
        n180 = property on="Holding Current" class="WFGraph (엄격한)"(error in=w455, "Active Cursor"=w459, "Cursor.Cursor X"=w460) -> (error out=w458:errorcluster)  [unwired: 1 in, 1 out]
        n181 = property on="Averaged Amplitude" class="WFGraph (엄격한)"(error in=w455, "Active Cursor"=w459, "Cursor.Cursor X"=w460) -> (error out=w457:errorcluster)  [unwired: 1 in, 1 out]
        n182 = property on="Number of event" class="WFGraph (엄격한)"(error in=w455, "Active Cursor"=w459, "Cursor.Cursor X"=w460) -> (error out=w456:errorcluster)  [unwired: 1 in, 1 out]
        n183 = Merge Errors(w458, w457, w456) -> (w454:errorcluster)
        n184 = call <vilib>:"Add State(s) to Queue__JKI_lib_State_Machine.vi"("State(s) in (\"\")"=w463) -> ("States Out"=w462:string)  [unwired: 14 in]
      }
      frame "UI: Update History log" {
        # "Do not put any code in this frame.\n(It is a separator no-op. You can make a copy of this frame to create a new UI frame)"
        n185 = Unbundle By Name(w475) -> ("History log"=w470:string, "Parameters.File.File Path"=w471:path, "Summary table"=w467:T11, "Parameters.Event Detection"=w466:T18, "Parameters.Smoothing"=w465:T2, "Sweep Num"=w464:u16)
        n186 = case shown="\"Import File\"" w472 {
          tunnel: w471 -> [_ _ _ _ _ w503 w510 _ _ _]
          tunnel: ["Minhee Analysis is initialized" "The data has been copied to the clipboard." "Unit file has been saved." "Whole result has been saved." "Analysis log has been saved." w502 w509 w535 w550 w568] -> w469
          tunnel: w467 -> [_ _ _ _ _ _ _ _ w547 w566]
          tunnel: w466 -> [_ _ _ _ _ w500 _ w533 _ _]
          tunnel: w465 -> [_ _ _ _ _ w499 _ w532 _ _]
          tunnel: w464 -> [_ _ _ _ _ _ _ w515 _ _]
          frame "Initialize", Default {
          }
          frame "Clipboard" {
          }
          frame "Save Unit File" {
          }
          frame "Save Whole Result" {
          }
          frame "Analysis Log" {
          }
          frame "Import initiallized" {
            n187 = Unbundle(w499) -> ("Polynomial order"=w492:i32, "Side points"=w491:i32)
            n188 = Unbundle(w500) -> ("Event threshold (amplitude)"=w498:dbl, "Polarity"=w495:T1)
            n189 = Number To Decimal String(number=w492) -> (decimal integer string=w490:string)  [unwired: 1 in]
            n190 = Number To Decimal String(number=w491) -> (decimal integer string=w488:string)  [unwired: 1 in]
            n191 = Number To Decimal String(number=w498) -> (decimal integer string=w497:string)  [unwired: 1 in]
            n192 = case shown="0, 기본" w495 {
              tunnel: ["Negative-going" ("문자열") "Positive-going" ("문자열")] -> w494
              frame 0, Default {
              }
              frame 1 {
              }
            }
            n193 = Path To String(path=w503) -> (string=w506:string)
            n194 = Concatenate Strings("Event detection is processing. (file: ", w506, ")", "\r", "\t", "Event Detection Parameters: Amplitude " ("문자열"), w497, " pA, " ("문자열"), w494, "\r", "\t", "Smoothing Parameters: Polynomial order " ("문자열"), w490, " , Side points " ("문자열"), w488) -> (w502:string)
          }
          frame "Import File" {
            n195 = Path To String(path=w510) -> (string=w513:string)
            n196 = Concatenate Strings("File is imported. (File path: ", w513, ")") -> (w509:string)
          }
          frame "Redetect" {
            n197 = Number To Decimal String(number=w515) -> (decimal integer string=w514:string)  [unwired: 1 in]
            n198 = Unbundle(w532) -> ("Polynomial order"=w525:i32, "Side points"=w524:i32)
            n199 = Unbundle(w533) -> ("Event threshold (amplitude)"=w531:dbl, "Polarity"=w528:T1)
            n200 = Number To Decimal String(number=w525) -> (decimal integer string=w523:string)  [unwired: 1 in]
            n201 = Number To Decimal String(number=w524) -> (decimal integer string=w521:string)  [unwired: 1 in]
            n202 = Number To Decimal String(number=w531) -> (decimal integer string=w530:string)  [unwired: 1 in]
            n203 = case shown="0, 기본" w528 {
              tunnel: ["Negative going" ("문자열") "Positive going" ("문자열")] -> w527
              frame 0, Default {
              }
              frame 1 {
              }
            }
            n204 = Concatenate Strings("Events are redetecting in SWEEP NUMBER " ("문자열"), w514, ".", "\r", "\t", "Event Detection Parameters: Amplitude " ("문자열"), w530, " pA, " ("문자열"), w527, "\r", "\t", "Smoothing Parameters: Polynomial order " ("문자열"), w523, " , Side points " ("문자열"), w521) -> (w535:string)
          }
          frame "Import done" {
            w549 = "#######################################################################################" ("문자열")
            w542 = "\r"
            n205 = Unbundle By Name(w547) -> ("Total.Event Num"=w546:string, "Total.Amplitude"=w544:string, "Total.ISI"=w543:string, "Total.Frequency"=w541:string)
            n206 = Concatenate Strings("Detection is finished. " ("문자열"), w542, w549, w542, "#   Number of detected events: " ("문자열"), w546, ", Mean amplitude: " ("문자열"), w544, " pA, Mean IEI: " ("문자열"), w543, " sec, Mean Frequency: " ("문자열"), w541, " Hz    #" ("문자열"), w542, w549) -> (w550:string)
          }
          frame "Select" {
            w567 = "#######################################################################################" ("문자열")
            w561 = "\r"
            n207 = Unbundle By Name(w566) -> ("Selected.Event Num"=w565:string, "Selected.Amplitude"=w563:string, "Selected.ISI"=w562:string, "Selected.Frequency"=w560:string, "Selected.Begin (sec)"=w556:string, "Selected.End (sec)"=w554:string)
            n208 = Concatenate Strings("Events between " ("문자열"), w556, " (sec) and " ("문자열"), w554, " (sec) are selected. " ("문자열"), w561, w567, w561, "#   Number of selected events: " ("문자열"), w565, ", Mean amplitude: " ("문자열"), w563, " pA, Mean IEI: " ("문자열"), w562, " sec, Mean Frequency: " ("문자열"), w560, " Hz    #" ("문자열"), w561, w567) -> (w568:string)
          }
        }
        n209 = call "History log.vi"("Message"=w469, "String IN"=w470) -> ("String OUT"=w473:string)  [unwired: 5 in]
        "History log" <- w473
        n210 = property on="History log" class="Str"("Text.Scroll Position"=u32 4294967295 ("텍스트.스크롤 위치")) -> ()  [unwired: 2 in, 2 out]
        n211 = Bundle By Name(cluster=w475, "History log"=w473) -> (w474:T9)
        n212 = call <vilib>:"Add State(s) to Queue__JKI_lib_State_Machine.vi"("State(s) in (\"\")"=w478) -> ("States Out"=w477:string)  [unwired: 14 in]
      }
      frame "UI: Cursor Set" {
        # "Argument"
        # "Set and Unset Cursor Busy.\n(Usage: \"UI: Cursor Set >> Busy|Idle\")"
        n213 = case shown="\"Idle\", 기본" w571 {
          tunnel: w573 -> [w578 w580]
          tunnel: [w577 w579] -> w572
          frame "Idle", Default {
            n214 = call <vilib>:"Unset Busy.vi"("error in (no error)"=w578) -> ("error out"=w577:errorcluster)  [unwired: 10 in]
          }
          frame "Busy" {
            n215 = call <vilib>:"Set Busy.vi"("error in (no error)"=w580) -> ("error out"=w579:errorcluster)  [unwired: 9 in, 1 out]
          }
        }
        n216 = call <vilib>:"Add State(s) to Queue__JKI_lib_State_Machine.vi"("State(s) in (\"\")"=w576) -> ("States Out"=w575:string)  [unwired: 14 in]
      }
      frame "UI: Front Panel State" {
        # "Argument"
        # "Set Front Panel Open or Closed\n(Usage: \"UI: Front Panel State >> Open|Close\")"
        n217 = Unbundle By Name(w583) -> ("Core.Current VI Reference"=w582:refnum<vi>)
        n218 = case shown="\"Open\", \"Standard\", 기본" w581 {
          tunnel: w585 -> [w593 w608 w619 w632 w645]
          tunnel: [w595 w609 w621 w634 w647] -> w584
          tunnel: w582 -> [w594 w606 w620 w633 w646]
          frame "Open", "Standard", Default {
            w588 = T4."Standard" ("State")
            n219 = property class="VI"(reference=w594, error in=w593) -> (reference out=w591:refnum<vi>, error out=w592:errorcluster, "FP.State"=w590:T4)
            n220 = Not Equal?(x=w590, y=w588) -> (x != y?=w589:bool)
            n221 = case shown="참" w589 {
              tunnel: [w599 w601] -> w595
              tunnel: w592 -> [w598 w601]
              tunnel: w591 -> [w597 _]
              tunnel: w588 -> [w596 _]
              frame True {
                n222 = invoke class="VI" method="FP.Open"(reference=w597, error in=w598, "Activate"=TRUE, "State"=w596) -> (error out=w599:errorcluster)  [unwired: 1 in, 4 out]
              }
              frame False {
              }
            }
          }
          frame "Close", "Closed" {
            n223 = property class="VI"(reference=w606, error in=w608) -> (reference out=w605:refnum<vi>, error out=w607:errorcluster, "FP.State"=w603:T4)
            n224 = Not Equal?(x=w603, y=T4."Closed" ("Front Panel Window:State")) -> (x != y?=w602:bool)
            n225 = case shown="참" w602 {
              tunnel: [w610 w613] -> w609
              tunnel: w607 -> [w610 w612]
              tunnel: w605 -> [_ w611]
              frame False {
              }
              frame True {
                n226 = invoke class="VI" method="FP.Close"(reference=w611, error in=w612) -> (error out=w613:errorcluster)  [unwired: 1 in, 2 out]
              }
            }
          }
          frame "Hidden", "Hide" {
            w614 = T4."Hidden" ("State")
            n227 = property class="VI"(reference=w620, error in=w619) -> (reference out=w617:refnum<vi>, error out=w618:errorcluster, "FP.State"=w616:T4)
            n228 = Not Equal?(x=w616, y=w614) -> (x != y?=w615:bool)
            n229 = case shown="참" w615 {
              tunnel: [w625 w626] -> w621
              tunnel: w618 -> [w624 w626]
              tunnel: w617 -> [w623 _]
              tunnel: w614 -> [w622 _]
              frame True {
                n230 = invoke class="VI" method="FP.Open"(reference=w623, error in=w624, "State"=w622) -> (error out=w625:errorcluster)  [unwired: 2 in, 4 out]
              }
              frame False {
              }
            }
          }
          frame "Minimize", "Minimized" {
            w627 = T4."Minimized" ("State")
            n231 = property class="VI"(reference=w633, error in=w632) -> (reference out=w630:refnum<vi>, error out=w631:errorcluster, "FP.State"=w629:T4)
            n232 = Not Equal?(x=w629, y=w627) -> (x != y?=w628:bool)
            n233 = case shown="참" w628 {
              tunnel: [w638 w639] -> w634
              tunnel: w631 -> [w637 w639]
              tunnel: w630 -> [w636 _]
              tunnel: w627 -> [w635 _]
              frame True {
                n234 = invoke class="VI" method="FP.Open"(reference=w636, error in=w637, "State"=w635) -> (error out=w638:errorcluster)  [unwired: 2 in, 4 out]
              }
              frame False {
              }
            }
          }
          frame "Maximize", "Maximized" {
            w640 = T4."Maximized" ("State")
            n235 = property class="VI"(reference=w646, error in=w645) -> (reference out=w643:refnum<vi>, error out=w644:errorcluster, "FP.State"=w642:T4)
            n236 = Not Equal?(x=w642, y=w640) -> (x != y?=w641:bool)
            n237 = case shown="참" w641 {
              tunnel: [w651 w652] -> w647
              tunnel: w644 -> [w650 w652]
              tunnel: w643 -> [w649 _]
              tunnel: w640 -> [w648 _]
              frame True {
                n238 = invoke class="VI" method="FP.Open"(reference=w649, error in=w650, "State"=w648) -> (error out=w651:errorcluster)  [unwired: 2 in, 4 out]
              }
              frame False {
              }
            }
          }
        }
        n239 = call <vilib>:"Add State(s) to Queue__JKI_lib_State_Machine.vi"("State(s) in (\"\")"=w587) -> ("States Out"=w586:string)  [unwired: 14 in]
      }
      frame "---------- Macro ----------" {
        # "Do not put any code in this frame.\n(It is a separator no-op. You can make a copy of this frame to create a new Macro frame)"
        n240 = call <vilib>:"Add State(s) to Queue__JKI_lib_State_Machine.vi"("State(s) in (\"\")"=w656) -> ("States Out"=w655:string)  [unwired: 14 in]
      }
      frame "Macro: Initialize" {
        w657 = "Data: Initialize\nInitialize Core Data\nUI: Initialize \nMacro: Initialize UI\nData: Insert inital parameters\nUI: Front Panel State >> Open \nUI: Update History log >> Initialize"  # Data: Initialize Initialize Core Data UI: Initialize  Macro: Initialize UI Data: Insert inital parameters UI: Front Panel State >> Open  UI: Update History log >> Initialize
        # "Initialization Macro\n(This is called once, when the VI starts)"
        n241 = call <vilib>:"Add State(s) to Queue__JKI_lib_State_Machine.vi"("State(s) in Front (\"\")"=w657, "State(s) in (\"\")"=w661) -> ("States Out"=w660:string)  [unwired: 13 in]
      }
      frame "Macro: Initialize UI" {
        # "Initialization Macro\n(This is called once, when the VI starts)"
        n242 = call <vilib>:"Add State(s) to Queue__JKI_lib_State_Machine.vi"("State(s) in Front (\"\")"="UI: Update Whole trace\nUI: Update Whole trace cursor\nUI: Update Event trace \nUI: Update Sweep Info\nUI: Update Event Table \nUI: Update Total table\nUI: Update Selected table", "State(s) in (\"\")"=w666) -> ("States Out"=w665:string)  [unwired: 13 in]
      }
      frame "Macro: Update UI related with Sweep" {
        # "Initialization Macro\n(This is called once, when the VI starts)"
        n243 = call <vilib>:"Add State(s) to Queue__JKI_lib_State_Machine.vi"("State(s) in Front (\"\")"="UI: Update Whole trace \nUI: Update Event Table \nUI: Update Sweep infor cursor", "State(s) in (\"\")"=w671) -> ("States Out"=w670:string)  [unwired: 13 in]
      }
      frame "Macro: Update UI related with Event" {
        # "Initialization Macro\n(This is called once, when the VI starts)"
        n244 = call <vilib>:"Add State(s) to Queue__JKI_lib_State_Machine.vi"("State(s) in Front (\"\")"="UI: Update Event trace \nUI: Update Whole trace cursor", "State(s) in (\"\")"=w676) -> ("States Out"=w675:string)  [unwired: 13 in]
      }
      frame "Macro: Exit" {
        # "Exit Macro\n(This is called once, when the VI exits)"
        n245 = Unbundle By Name(w683) -> ("Core.Close Panel on Exit?"=w682:bool)
        n246 = Two Button Dialog(message="Are you sure you want to quit?" ("메시지"), 1:"Cancel" ("거짓 버튼 이름(\"취소\")"), 2:"Yes" ("참 버튼 이름(\"확인\")")) -> (T button?=w678:bool)
        n247 = case shown="거짓" w678 {
          tunnel: w682 -> [_ w693]
          tunnel: ["" ("States Out") w688] -> w681
          frame False {
          }
          frame True {
            n248 = Select(t="UI: Front Panel State >> Close", s=w693, f="") -> (s? t:f=w690:string)
            n249 = call <vilib>:"Add State(s) to Queue__JKI_lib_State_Machine.vi"("State(s) in (\"\")"=w690, "State(s) at Back (\"\")"="Data: Cleanup\nExit") -> ("States Out"=w688:string)  [unwired: 13 in]
          }
        }
        n250 = call <vilib>:"Add State(s) to Queue__JKI_lib_State_Machine.vi"("State(s) in Front (\"\")"=w681, "State(s) in (\"\")"=w686) -> ("States Out"=w685:string)  [unwired: 13 in]
      }
      frame "---------- Action ----------" {
        # "Template Separator\n(You can make a copy of, or modify, this frame)"
        n251 = call <vilib>:"Add State(s) to Queue__JKI_lib_State_Machine.vi"("State(s) in (\"\")"=w697) -> ("States Out"=w696:string)  [unwired: 14 in]
      }
      frame "Action: Import ABF File" {
        # "Your code here.\n(You can make a copy of, or modify, this frame)"
        n252 = call "파일 대화 상자"("pattern (all files)"="*.abf") -> ("selected path"=w701:path, "error out"=w700:errorcluster)  [unwired: 11 in, 2 out]
        n253 = Merge Errors(w700, w699) -> (w698:errorcluster)
        n254 = call "ABF_Read.vi"("error in (no error)"=w698, "Path of ABF file"=w701) -> ("error out"=w707:errorcluster, "File Paramters"=w712:T19, "Whole Trace"=w715:sgl[][])  [unwired: 3 in]
        n255 = Unbundle(w712) -> ("File Name"=w711:string, "Total Length"=w710:i32, "Trial Length (ms)"=w709:dbl, "Sweep Number"=w705:dbl, "Sampling rate"=w708:dbl)  [unwired: 2 out]
        n256 = Decrement(x=w705) -> (x-1=w704:dbl)
        n257 = Bundle By Name(cluster=w714, "Whole trace (2D)"=w715, "Parameters.File.File Path"=w701, "Parameters.File.File Name"=w711, "Parameters.File.Total Length"=w710, "Parameters.File.Trial Length (ms)"=w709, "Parameters.File.Sweep Number"=w705, "Parameters.File.Sampling rate"=w708) -> (w713:T9)
        n258 = property on="Sweep Num" class="DigNum (엄격한)"(error in=w707, "Maximum"=w704, "Minimum"=0.0 ("데이터 입력 제한:최소")) -> (error out=w706:errorcluster)  [unwired: 1 in, 1 out]
        n259 = call <vilib>:"Add State(s) to Queue__JKI_lib_State_Machine.vi"("State(s) in (\"\")"=w717) -> ("States Out"=w716:string)  [unwired: 14 in]
      }
      frame "Action: Import DAT File" {
        # "Your code here.\n(You can make a copy of, or modify, this frame)"
        n260 = call "파일 대화 상자3"("pattern (all files)"="*.dat") -> ("selected path"=w727:path, "error out"=w729:errorcluster)  [unwired: 11 in, 2 out]
        n261 = Merge Errors(w729, w728) -> (w726:errorcluster)
        n262 = call "ReadHEKA.vi"("Error IN"=w726, "FilePath"=w727) -> ("Error OUT"=w725:errorcluster, "File Parameters"=w724:T20, "Traces"=w723:sgl[][])  [unwired: 7 in]
        n263 = Unbundle(w724) -> ("File name"=w722:string, "Total Length"=w721:i32, "Trial Length (ms)"=w720:i32, "Sweep Number"=w719:i32, "Sampling rate"=w718:dbl)  [unwired: 1 out]
        n264 = Decrement(x=w719) -> (x-1=w732:i32)
        n265 = Bundle By Name(cluster=w735, "Whole trace (2D)"=w723, "Parameters.File.File Path"=w727, "Parameters.File.File Name"=w722, "Parameters.File.Total Length"=w721, "Parameters.File.Trial Length (ms)"=w720, "Parameters.File.Sweep Number"=w719, "Parameters.File.Sampling rate"=w718) -> (w734:T9)
        n266 = property on="Sweep Num" class="DigNum (엄격한)"(error in=w725, "Maximum"=w732, "Minimum"=0.0 ("데이터 입력 제한:최소")) -> (error out=w733:errorcluster)  [unwired: 1 in, 1 out]
        n267 = call <vilib>:"Add State(s) to Queue__JKI_lib_State_Machine.vi"("State(s) in (\"\")"=w737) -> ("States Out"=w736:string)  [unwired: 14 in]
      }
      frame "Action: Import TXT File" {
        # "Your code here.\n(You can make a copy of, or modify, this frame)"
        n268 = call "파일 대화 상자2"("pattern (all files)"="*.txt") -> ("selected path"=w738:path)  [unwired: 11 in, 3 out]
        n269 = call "Additional config for txt file.vi"() -> ("Cancel"=w740:bool, "Configuration for text file"=w742:T21)  [unwired: 4 in]
        n270 = Unbundle By Name(w742) -> ("Sampling rate (Hz)"=w741:dbl)
        n271 = case shown="거짓" w740 {
          tunnel: [w766 _] -> w755
          tunnel: w738 -> [w765 _]
          tunnel: w742 -> [w764 _]
          tunnel: w741 -> [w763 _]
          tunnel: [w761 _] -> w752
          tunnel: [w760 w767] -> w747
          tunnel: w756 -> [w759 w767]
          frame False {
            n272 = call "TXT_Read.vi"("error in (no error)"=w759, "Configuration for text file"=w764, "Path of ABF file"=w765) -> ("error out"=w760:errorcluster, "File Paramters"=w762:T19, "Whole Trace"=w766:sgl[][])  [unwired: 1 in, 1 out]
            n273 = Bundle By Name(cluster=w762, "Sampling rate"=w763) -> (w761:T19)
          }
          frame True {
          }
        }
        n274 = Unbundle(w752) -> ("File Name"=w751:string, "Total Length"=w750:i32, "Trial Length (ms)"=w749:dbl, "Sweep Number"=w745:dbl, "Sampling rate"=w748:dbl)  [unwired: 2 out]
        n275 = Decrement(x=w745) -> (x-1=w744:dbl)
        n276 = Bundle By Name(cluster=w754, "Whole trace (2D)"=w755, "Parameters.File.File Path"=w738, "Parameters.File.File Name"=w751, "Parameters.File.Total Length"=w750, "Parameters.File.Trial Length (ms)"=w749, "Parameters.File.Sweep Number"=w745, "Parameters.File.Sampling rate"=w748) -> (w753:T9)
        n277 = property on="Sweep Num" class="DigNum (엄격한)"(error in=w747, "Maximum"=w744, "Minimum"=0.0 ("데이터 입력 제한:최소")) -> (error out=w746:errorcluster)  [unwired: 1 in, 1 out]
        n278 = call <vilib>:"Add State(s) to Queue__JKI_lib_State_Machine.vi"("State(s) in (\"\")"=w758) -> ("States Out"=w757:string)  [unwired: 14 in]
      }
      frame "Action: Event detection" {
        # "Sweep trace (2D) \n1. event point\n2. filtered trace\n3. trend\n4. raw trace"
        # "Your code here.\n(You can make a copy of, or modify, this frame)"
        n279 = Unbundle By Name(w804) -> ("Result.Detected Events (1D)"=w776:cluster{sgl[][]}[], "Result.Sweep Traces (2D)"=w779:cluster{sgl[], "X":sgl[]}[][], "Parameters"=w797:T7, "Whole trace (2D)"=w811:sgl[][], "Parameters.File.Sampling rate"=w809:dbl, "Parameters.Event Detection.Polarity"=w808:T1, "Parameters.File.Trial Length (ms)"=w807:dbl, "Parameters.Smoothing"=w773:T2, "Running Sweep Num"=w772:i32, "Parameters.File.Sweep Number"=w792:dbl, "Aborted?"=w791:bool, "Sweep Info.Averaged Amplitude"=w787:sgl[], "Sweep Info.Number of event"=w788:i32[], "Sweep Info.Holding Current"=w780:sgl[], "Smoothing Parameters (1D)"=w771:T10)
        n280 = Unbundle(w773) -> ("Polynomial order"=w805:i32, "Side points"=w806:i32)
        n281 = Index Array(array=w811, index (row)=w772) -> (element=w810:sgl[])  [unwired: 1 in]
        n282 = case shown="0, 기본" w808 {
          tunnel: [w821 w823] -> w817
          tunnel: [w820 w822] -> w814
          frame 0, Default {
            w820 = -3.0  # Threshold
            w821 = u16 1 items=["peaks", "valleys"] ("peaks/valleys")
          }
          frame 1 {
            w822 = 3.0  # Threshold
            w823 = u16 0 items=["peaks", "valleys"] ("peaks/valleys")
          }
        }
        n283 = call-poly <vilib>:"Savitzky-Golay Filter.vi"("polynomial order"=w805, "side points"=w806, "X"=w810) -> ("Filtered X"=w769:dbl[])  [unwired: 7 in, 1 out]
        n284 = Divide(x=w807, y=w809) -> (x/y=w816:dbl)
        n285 = To Single Precision Float(number=w769) -> (single precision float=w768:sgl[])
        n286 = Multiply(x=w816, y=w772) -> (x*y=w815:dbl)
        n287 = call "[Stepwise] Initial search.vi"("peaks/valleys"=w817, "숫자형"=w815, "Sampling rate"=w809, "에러 입력(에러 없음)"=w813, "Filtered X"=w768, "Whole trace (2D)"=w810, "Threshold"=w814) -> ("에러 출력"=w812:errorcluster, "Detected Event"=w801:cluster{dbl[][]}, "Initial Search"=w802:cluster{dbl[], "X":dbl[]}[])  [unwired: 1 in, 1 out]
        n288 = call "[Stepwise] Baseline calculation.vi"("Parameter IN"=w797, "Sweep trace (2D) IN"=w802, "Detected Event IN"=w801, "Running Sweep #"=w772) -> ("I hold"=w781:dbl, "Sweep trace (2D) OUT"=w800:cluster{"Ramp Pattern":dbl[], "X":dbl[]}[], "Detected Event OUT"=w799:cluster{dbl[][]}, "New Baseline OUT"=w798:cluster{dbl[][]})  [unwired: 2 in]
        n289 = call "[Stepwise] Final search.vi"("Parameter IN"=w797, "Sweep trace (2D) IN"=w800, "Detected Event IN"=w799, "Baseline infor IN"=w798) -> ("Mean Amplitude"=w785:dbl, "Number of EVT"=w786:i32, "Sweep trace (2D) OUT"=w778:cluster{"Ramp Pattern":dbl[], "X":dbl[]}[], "Detected Event OUT"=w775:cluster{dbl[][]})  [unwired: 2 in]
        n290 = Insert Into Array(array=w776, index=w772, new element=w775) -> (w774:cluster{sgl[][]}[])
        n291 = Insert Into Array(array=w779, index (row)=w772, new element=w778) -> (w777:cluster{sgl[], "X":sgl[]}[][])  [unwired: 1 in]
        n292 = Insert Into Array(array=w788, index=w772, new element=w786) -> (w783:i32[])
        n293 = Insert Into Array(array=w780, index=w772, new element=w781) -> (w782:sgl[])
        n294 = Insert Into Array(array=w787, index=w772, new element=w785) -> (w784:sgl[])
        n295 = Increment(x=w772) -> (x+1=w796:i32)
        n296 = Insert Into Array(array=w771, index=w772, new element=w773) -> (w770:T10)
        n297 = Bundle By Name(cluster=w804, "Result.Sweep Traces (2D)"=w777, "Running Sweep Num"=w796, "Sweep Info.Averaged Amplitude"=w784, "Sweep Info.Number of event"=w783, "Sweep Info.Holding Current"=w782, "Result.Detected Events (1D)"=w774, "Smoothing Parameters (1D)"=w770) -> (w803:T9)
        n298 = Greater Or Equal?(x=w796, y=w792) -> (x >= y?=w790:bool)
        n299 = Or(x=w790, y=w791) -> (x .or. y?=w789:bool)
        n300 = Select(t="Data: Whole trace selection\nUI: Update Sweep Info \nUI: Update Total table\nData: Insert Sweep num \nMacro: Update UI related with Sweep \nData: Insert Event num \nMacro: Update UI related with Event\nUI: Update History log >> Import done", s=w789, f="Event Structure \nUI: Update Sweep Info\nAction: Event detection") -> (s? t:f=w793:string)
        n301 = call <vilib>:"Add State(s) to Queue__JKI_lib_State_Machine.vi"("State(s) in Front (\"\")"=w793, "State(s) in (\"\")"=w819) -> ("States Out"=w818:string)  [unwired: 13 in]
      }
      frame "Action: Abort" {
        # "Template Separator\n(You can make a copy of, or modify, this frame)"
        n302 = Bundle By Name(cluster=w826, "Aborted?"=TRUE ("Aborted")) -> (w825:T9)
        n303 = call <vilib>:"Add State(s) to Queue__JKI_lib_State_Machine.vi"("State(s) in (\"\")"=w829) -> ("States Out"=w828:string)  [unwired: 14 in]
      }
      frame "Action: Redetect" {
        # "Template Separator\n(You can make a copy of, or modify, this frame)"
        n304 = Unbundle By Name(w847) -> ("Parameters"=w858:T7, "Whole trace (2D)"=w857:sgl[][], "Sweep Num"=w836:u16, "Result.Sweep Traces (2D)"=w845:cluster{sgl[], "X":sgl[]}[][], "Result.Detected Events (1D)"=w842:cluster{sgl[][]}[], "Sweep Info.Averaged Amplitude"=w839:sgl[], "Sweep Info.Number of event"=w837:i32[])
        n305 = Index Array(array=w857, index (row)=w836) -> (element=w856:sgl[])  [unwired: 1 in]
        n306 = call "[Redetection] initial search.vi"("error in (no error)"=w831, "Sweep #"=w836, "Data (1 sweep)"=w856, "Parameter setting IN"=w858) -> ("error out"=w852:errorcluster, "Sweep trace"=w853:cluster{dbl[], "X":dbl[]}[], "Detected event"=w854:cluster{dbl[][]}, "Parameter setting OUT"=w855:T7)  [unwired: 4 in]
        n307 = call "[Redetection] Baseline calculation.vi"("Sweep #"=w836, "error in (no error)"=w852, "Sweep trace (1D)"=w853, "Detected event"=w854, "Parameter setting IN"=w855) -> ("error out"=w830:errorcluster, "Sweep trace (1D) OUT"=w849:cluster{"Ramp Pattern":dbl[], "X":dbl[]}[], "Detected event OUT"=w850:cluster{dbl[][]}, "New baseline info"=w851:cluster{dbl[][]}, "Parameter setting OUT"=w848:T7)  [unwired: 2 in]
        n308 = call "[Redetection] Final Search.vi"("Parameter setting IN"=w848, "Sweep trace (1D) IN"=w849, "Detected event IN"=w850, "New baseline info IN"=w851) -> ("Number of redetected evt"=w835:i32, "Sweep trace (1D) Out"=w844:cluster{"Ramp Pattern":dbl[], "X":dbl[]}[], "Mean Amplitude of retected evt"=w838:dbl, "Detected Event OUT"=w840:cluster{dbl[][]})  [unwired: 3 in]
        n309 = Replace Array Subset(array=w842, new element=w840, index=w836) -> (w841:cluster{sgl[][]}[])
        n310 = Replace Array Subset(array=w839, new element=w838, index=w836) -> (w834:sgl[])
        n311 = Replace Array Subset(array=w837, new element=w835, index=w836) -> (w833:i32[])
        n312 = Replace Array Subset(array=w845, new element=w844, index (row)=w836) -> (w843:cluster{sgl[], "X":sgl[]}[][])  [unwired: 1 in]
        n313 = Bundle By Name(cluster=w847, "Result.Sweep Traces (2D)"=w843, "Result.Detected Events (1D)"=w841, "Sweep Info.Averaged Amplitude"=w834, "Sweep Info.Number of event"=w833) -> (w846:T9)
        n314 = call <vilib>:"Add State(s) to Queue__JKI_lib_State_Machine.vi"("State(s) in Front (\"\")"="UI: Update Sweep Info \nUI: Update Total table\nData: Insert Sweep num \nMacro: Update UI related with Sweep \nData: Insert Event num \nMacro: Update UI related with Event \nUI: Update History log >> Redetect \nUI: Update History log >> Import done", "State(s) in (\"\")"=w860) -> ("States Out"=w859:string)  [unwired: 13 in]
      }
      frame "Action: Delete" {
        # "Template Separator\n(You can make a copy of, or modify, this frame)"
        n315 = Unbundle By Name(w880) -> ("Result.Detected Events (1D)"=w876:cluster{sgl[][]}[], "Result.Sweep Traces (2D)"=w877:cluster{sgl[], "X":sgl[]}[][], "Sweep Num"=w862:u16, "Event Num"=w875:i16, "Sweep Info.Averaged Amplitude"=w863:sgl[], "Sweep Info.Number of event"=w866:i32[])  [unwired: 2 out]
        n316 = call "[Delete] Main.vi"("Event #"=w875, "error in (no error)"=w872, "Sweep #"=w862, "Sweep trace (2D) IN"=w877, "Detected Event (1D) IN"=w876) -> ("error out"=w871:errorcluster, "부분이 삭제된 배열"=w870:dbl[][], "Sweep trace (2D) Out"=w874:cluster{"Ramp Pattern":dbl[], "X":dbl[]}[][], "Detected Event (1D) Out"=w873:cluster{dbl[][]}[])
        n317 = Index Array(array=w870, index (col)=4 ("비활성화된 인덱스 (열)")) -> (element=w868:dbl[])  [unwired: 1 in]
        n318 = call <vilib>:"Std Deviation and Variance.vi"("X"=w868) -> ("mean"=w861:dbl)  [unwired: 1 in, 2 out]
        n319 = Array Size(array=w868) -> (size(s)=w865:i32)
        n320 = Replace Array Subset(array=w863, new element=w861, index=w862) -> (w864:sgl[])
        n321 = Replace Array Subset(array=w866, new element=w865, index=w862) -> (w867:i32[])
        n322 = Bundle By Name(cluster=w880, "Result.Detected Events (1D)"=w873, "Result.Sweep Traces (2D)"=w874, "Sweep Info.Averaged Amplitude"=w864, "Sweep Info.Number of event"=w867) -> (w879:T9)
        n323 = call <vilib>:"Add State(s) to Queue__JKI_lib_State_Machine.vi"("State(s) in Front (\"\")"="UI: Update Sweep Info \nUI: Update Total table\nData: Insert Sweep num \nMacro: Update UI related with Sweep \nData: Insert Event num \nMacro: Update UI related with Event \nUI: Update History log >> Redetect \nUI: Update History log >> Import done", "State(s) in (\"\")"=w882) -> ("States Out"=w881:string)  [unwired: 13 in]
      }
      frame "Action: Selection" {
        # "Template Separator\n(You can make a copy of, or modify, this frame)"
        n324 = Unbundle By Name(w904) -> ("Number of Event to select"=w909:i32, "Result.Detected Events (1D)"=w933:cluster{sgl[][]}[], "Sweep Num"=w930:u16, "Event Num"=w928:i16, "Sweep Info.Number of event"=w931:i32[])  [unwired: 1 out]
        n325 = Array Size(array=w933) -> (size(s)=w934:i32)
        n326 = Split 1D Array(array=w931, index=w930) -> (first subarray=w929:i32[], second subarray=w911:i32[])
        n327 = for {
          N: w934 -> [_]
          shift-right: [w952] -> _
          shift-left: w933 -> [w952]
          shift-right: [w950] -> w907
          shift-left: sgl[][] [] -> [w949]
          i -> [w948]
          n328 = Index Array(array=w952, index=w948) -> (element=w951:cluster{sgl[][]})
          n329 = Unbundle(w951) -> (w947:sgl[][])
          n330 = Insert Into Array(array=w949, new element=w947) -> (w950:sgl[][])  [unwired: 2 in]
        }
        n331 = Add Array Elements(numeric array=w929) -> (sum=w927:i32)
        n332 = Add Array Elements(numeric array=w911) -> (sum=w908:i32)
        n333 = Add(x=w928, y=w927) -> (x+y=w906:i32)
        n334 = Array Size(array=w907) -> (size(s)=w926:i32[])
        n335 = Greater Or Equal?(x=w908, y=w909) -> (x >= y?=w910:bool)
        n336 = case shown="거짓" w910 {
          tunnel: w909 -> [_ w940]
          tunnel: [w939 w940] -> w893
          tunnel: w908 -> [w939 _]
          frame False {
          }
          frame True {
          }
        }
        n337 = Index Array(array=w926) -> (element=w925:i32)  [unwired: 1 in]
        n338 = Initialize Array(0.0 ("원소"), w925) -> (w921:dbl[])
        n339 = Initialize Array(1.0 ("원소"), w893) -> (w920:dbl[])
        n340 = Number To Decimal String(number=w893) -> (decimal integer string=w902:string)  [unwired: 1 in]
        n341 = Delete From Array(array=w907, length=w893, index (row)=w906) -> (deleted portion=w905:sgl[][])  [unwired: 1 in, 1 out]
        n342 = Replace Array Subset(array=w921, new element=w920, index=w906) -> (w885:dbl[])
        n343 = Index Array(array=w905, index (col) #1=4 ("비활성화된 인덱스 (열)"), index (col) #2=2 ("인덱스 (열)")) -> (element #1=w913:sgl[], element #2=w899:sgl[])  [unwired: 2 in]
        n344 = To Single Precision Float(number=w885) -> (single precision float=w884:sgl[])
        n345 = Decrement(x=w893) -> (x-1=w897:i32)
        n346 = call <vilib>:"Std Deviation and Variance.vi"("X"=w913) -> ("mean"=w915:dbl)  [unwired: 1 in, 2 out]
        n347 = Replace Array Subset(array=w907, new element=w884, index (col)=5 ("비활성화된 인덱스 (열)")) -> (w883:sgl[][])  [unwired: 1 in]
        n348 = for {
          N: w897 -> [_]
          tunnel: [w944] -> w917 mode=indexing
          tunnel: w899 -> [w943]
          i -> [w945]
          n349 = Increment(x=w945) -> (x+1=w946:i32)
          n350 = Index Array(array=w943, index #1=w946, index #2=w945) -> (element #1=w942:sgl, element #2=w941:sgl)
          n351 = Subtract(x=w942, y=w941) -> (x-y=w944:sgl)
        }
        n352 = Index Array(array=w899, index #1=0 ("인덱스"), index #2=w897) -> (element #1=w889:sgl, element #2=w888:sgl)
        n353 = Number To Fractional String(number=w915, precision (6)=i16 2 ("폭(-)")) -> (F-format string=w901:string)  [unwired: 2 in]
        n354 = Subtract(x=w888, y=w889) -> (x-y=w892:sgl)
        n355 = Divide(x=w893, y=w892) -> (x/y=w895:sgl)
        n356 = Number To Fractional String(number=w889, precision (6)=i16 3 ("폭(-)")) -> (F-format string=w887:string)  [unwired: 2 in]
        n357 = Number To Fractional String(number=w888, precision (6)=i16 3 ("폭(-)")) -> (F-format string=w886:string)  [unwired: 2 in]
        n358 = call <vilib>:"Std Deviation and Variance.vi"("X"=w917) -> ("mean"=w919:dbl)  [unwired: 1 in, 2 out]
        n359 = Number To Fractional String(number=w895, precision (6)=i16 3 ("폭(-)")) -> (F-format string=w894:string)  [unwired: 2 in]
        n360 = Number To Fractional String(number=w919, precision (6)=i16 2 ("폭(-)")) -> (F-format string=w900:string)  [unwired: 2 in]
        n361 = Bundle By Name(cluster=w904, "Final Data"=w883, "Summary table.Selected.Event Num"=w902, "Summary table.Selected.Amplitude"=w901, "Summary table.Selected.ISI"=w900, "Summary table.Selected.Frequency"=w894, "Summary table.Selected.Begin (sec)"=w887, "Summary table.Selected.End (sec)"=w886) -> (w903:T9)
        n362 = call <vilib>:"Add State(s) to Queue__JKI_lib_State_Machine.vi"("State(s) in Front (\"\")"="UI: Update Selected table \nUI: Update History log >> Select ", "State(s) in (\"\")"=w938) -> ("States Out"=w937:string)  [unwired: 13 in]
      }
      frame "Action: File Explorer" {
        # "Template Separator\n(You can make a copy of, or modify, this frame)"
        n363 = Unbundle By Name(w954) -> ("Parameters.File.File Path"=w953:path)
        n364 = call <vilib>:"Show in File System.vi"("error in (no error)"=w956, "file or directory path"=w953) -> ("error out"=w955:errorcluster)  [unwired: 9 in]
        n365 = call <vilib>:"Add State(s) to Queue__JKI_lib_State_Machine.vi"("State(s) in (\"\")"=w958) -> ("States Out"=w957:string)  [unwired: 14 in]
      }
      frame "Action: Clipboard" {
        # "Template Separator\n(You can make a copy of, or modify, this frame)"
        n366 = Unbundle By Name(w965) -> ("Final Data"=w960:sgl[][])
        n367 = Number To Exponential String(number=w960) -> (E-format string=w961:string[][])  [unwired: 3 in]
        n368 = call <userlib>:"Clipboard transformation.vi"("Input (structured)"=w961) -> ("Output (flattened)"=w962:string)  [unwired: 1 in, 1 out]
        n369 = Open Application Reference() -> (0:w964:errorcluster)  [unwired: 4 in, 1 out]
        n370 = invoke class="App" method="Clipboard.Write"(error in=w964, "Param 0"=w962) -> (reference out=w963:refnum<vi>)  [unwired: 2 in, 3 out]
        n371 = Close Reference(reference=w963) -> ()  [unwired: 1 in, 1 out]
        n372 = call <vilib>:"Add State(s) to Queue__JKI_lib_State_Machine.vi"("State(s) in Front (\"\")"="UI: Update History log >> Clipboard", "State(s) in (\"\")"=w968) -> ("States Out"=w967:string)  [unwired: 13 in]
      }
      frame "Action: Save Unit File" {
        # "Template Separator\n(You can make a copy of, or modify, this frame)"
        n373 = Unbundle By Name(w982) -> ("Final Data"=w981:sgl[][])  [unwired: 1 out]
        n374 = Index Array(array=w981, index (col) #1=2 ("비활성화된 인덱스 (열)"), index (col) #2=4 ("인덱스 (열)"), index (col) #3=5 ("인덱스 (열)")) -> (element #1=w977:sgl[], element #2=w976:sgl[], element #3=w975:sgl[])  [unwired: 3 in]
        n375 = Build Array(w977, w976, w975) -> (w974:sgl[][])
        n376 = Transpose 2D Array(2D array=w974) -> (transposed array=w973:sgl[][])
        n377 = call-poly <vilib>:"Write Delimited Spreadsheet.vi"("format (%.3f)"="%.5f", "2D data"=w973, "error in (no error)"=w970, "transpose? (no:F)"=FALSE ("transpose? (F)")) -> ("error out"=w969:errorcluster)  [unwired: 10 in, 1 out]
        n378 = call <vilib>:"Add State(s) to Queue__JKI_lib_State_Machine.vi"("State(s) in Front (\"\")"="UI: Update History log >> Save Unit File", "State(s) in (\"\")"=w985) -> ("States Out"=w984:string)  [unwired: 13 in]
      }
      frame "Action: Save Whole Result" {
        # "Template Separator\n(You can make a copy of, or modify, this frame)"
        n379 = Unbundle By Name(w993) -> ("Final Data"=w989:sgl[][])  [unwired: 1 out]
        n380 = Number To Fractional String(number=w989) -> (F-format string=w988:string[][])  [unwired: 3 in]
        n381 = Build Array (concatenate)(string[] ["Baseline X (sec)", "Baseline Y (pA)", "Event X (sec)", "Event Y (pA)", "Amplitude (pA)", "Selection Index"], w988) -> (w986:string[][])
        n382 = call-poly <vilib>:"Write Delimited Spreadsheet.vi"("2D data"=w986, "error in (no error)"=w991, "transpose? (no:F)"=FALSE ("transpose? (F)")) -> ("error out"=w990:errorcluster)  [unwired: 11 in, 1 out]
        n383 = call <vilib>:"Add State(s) to Queue__JKI_lib_State_Machine.vi"("State(s) in Front (\"\")"="UI: Update History log >> Save Whole Result", "State(s) in (\"\")"=w996) -> ("States Out"=w995:string)  [unwired: 13 in]
      }
      frame "Action: Save History Log" {
        # "Template Separator\n(You can make a copy of, or modify, this frame)"
        n384 = Unbundle By Name(w1002) -> ("History log"=w998:string)
        n385 = call <userlib>:"FlattenedStructured.vi"("Input (flattened)"=w998) -> ("Output (stuctured)"=w997:string[][])  [unwired: 1 in, 1 out]
        n386 = call-poly <vilib>:"Write Delimited Spreadsheet.vi"("2D data"=w997, "error in (no error)"=w1000, "transpose? (no:F)"=FALSE ("transpose? (F)")) -> ("error out"=w999:errorcluster)  [unwired: 11 in, 1 out]
        n387 = call <vilib>:"Add State(s) to Queue__JKI_lib_State_Machine.vi"("State(s) in Front (\"\")"="UI: Update History log >> Analysis Log", "State(s) in (\"\")"=w1005) -> ("States Out"=w1004:string)  [unwired: 13 in]
      }
    }
  }
